vi "ゲージデータ取り込み.vi"(8 "測定周期/ms":dbl, 9 "値転記用配列_\n設定項目画面からの転記":T1[](array[typedef]) {"測定モード" items=["単発測定モード", "連続測定モード", "多点測定モード"]}, 10 "ゲージ確認ボタンBOOL":bool) -> (0 "書込周期/ms":dbl, 11 "実測設定項目配列_\nメインからの転記":T1[](array[typedef]) {"測定モード" items=["単発測定モード", "連続測定モード", "多点測定モード"]})   [LabVIEW 2021]
uses:
  <vilib>/Utility/config.llb/Read Key (U32).vi
  <vilib>/Utility/config.llb/Read Key (String).vi
  <vilib>/Utility/config.llb/Read Key (I32).vi
  <vilib>/Utility/config.llb/Read Key (Boolean).vi
  <vilib>/Utility/config.llb/NI_LVConfig.lvlib
panel:
  out "メイン設定_設定 12":T1 {"測定モード" items=["単発測定モード", "連続測定モード", "多点測定モード"]}
  out "メイン設定_設定 11":T1 {"測定モード" items=["単発測定モード", "連続測定モード", "多点測定モード"]}
  out "メイン設定_設定 10":T1 {"測定モード" items=["単発測定モード", "連続測定モード", "多点測定モード"]}
  out "メイン設定_設定 9":T1 {"測定モード" items=["単発測定モード", "連続測定モード", "多点測定モード"]}
  out "メイン設定_設定 8":T1 {"測定モード" items=["単発測定モード", "連続測定モード", "多点測定モード"]}
  out "メイン設定_設定 7":T1 {"測定モード" items=["単発測定モード", "連続測定モード", "多点測定モード"]}
  out "メイン設定_設定 6":T1 {"測定モード" items=["単発測定モード", "連続測定モード", "多点測定モード"]}
  out "メイン設定_設定 5":T1 {"測定モード" items=["単発測定モード", "連続測定モード", "多点測定モード"]}
  out "メイン設定_設定 4":T1 {"測定モード" items=["単発測定モード", "連続測定モード", "多点測定モード"]}
  out "メイン設定_設定 3":T1 {"測定モード" items=["単発測定モード", "連続測定モード", "多点測定モード"]}
  out "メイン設定_設定 2":T1 {"測定モード" items=["単発測定モード", "連続測定モード", "多点測定モード"]}
  out "メイン設定_設定 1":T1 {"測定モード" items=["単発測定モード", "連続測定モード", "多点測定モード"]}
  out "setup.iniエラーout":errorcluster caption="エラー入力（エラーなし）"
  out "iniフォルダパス取得":path
  in  "setup.iniエラーin":errorcluster caption="エラー入力（エラーなし）"
  out "ゲージエラー 12":errorcluster caption="エラー入力 (エラーなし)"
  out "ゲージエラー 11":errorcluster caption="エラー入力 (エラーなし)"
  out "ゲージエラー 10":errorcluster caption="エラー入力 (エラーなし)"
  out "ゲージエラー 9":errorcluster caption="エラー入力 (エラーなし)"
  out "ゲージエラー 8":errorcluster caption="エラー入力 (エラーなし)"
  out "ゲージエラー 7":errorcluster caption="エラー入力 (エラーなし)"
  out "ゲージエラー 6":errorcluster caption="エラー入力 (エラーなし)"
  out "ゲージエラー 5":errorcluster caption="エラー入力 (エラーなし)"
  out "ゲージエラー 4":errorcluster caption="エラー入力 (エラーなし)"
  out "ゲージエラー 3":errorcluster caption="エラー入力 (エラーなし)"
  out "ゲージエラー 2":errorcluster caption="エラー入力 (エラーなし)"
  out "ゲージエラー 1":errorcluster caption="エラー入力 (エラーなし)"
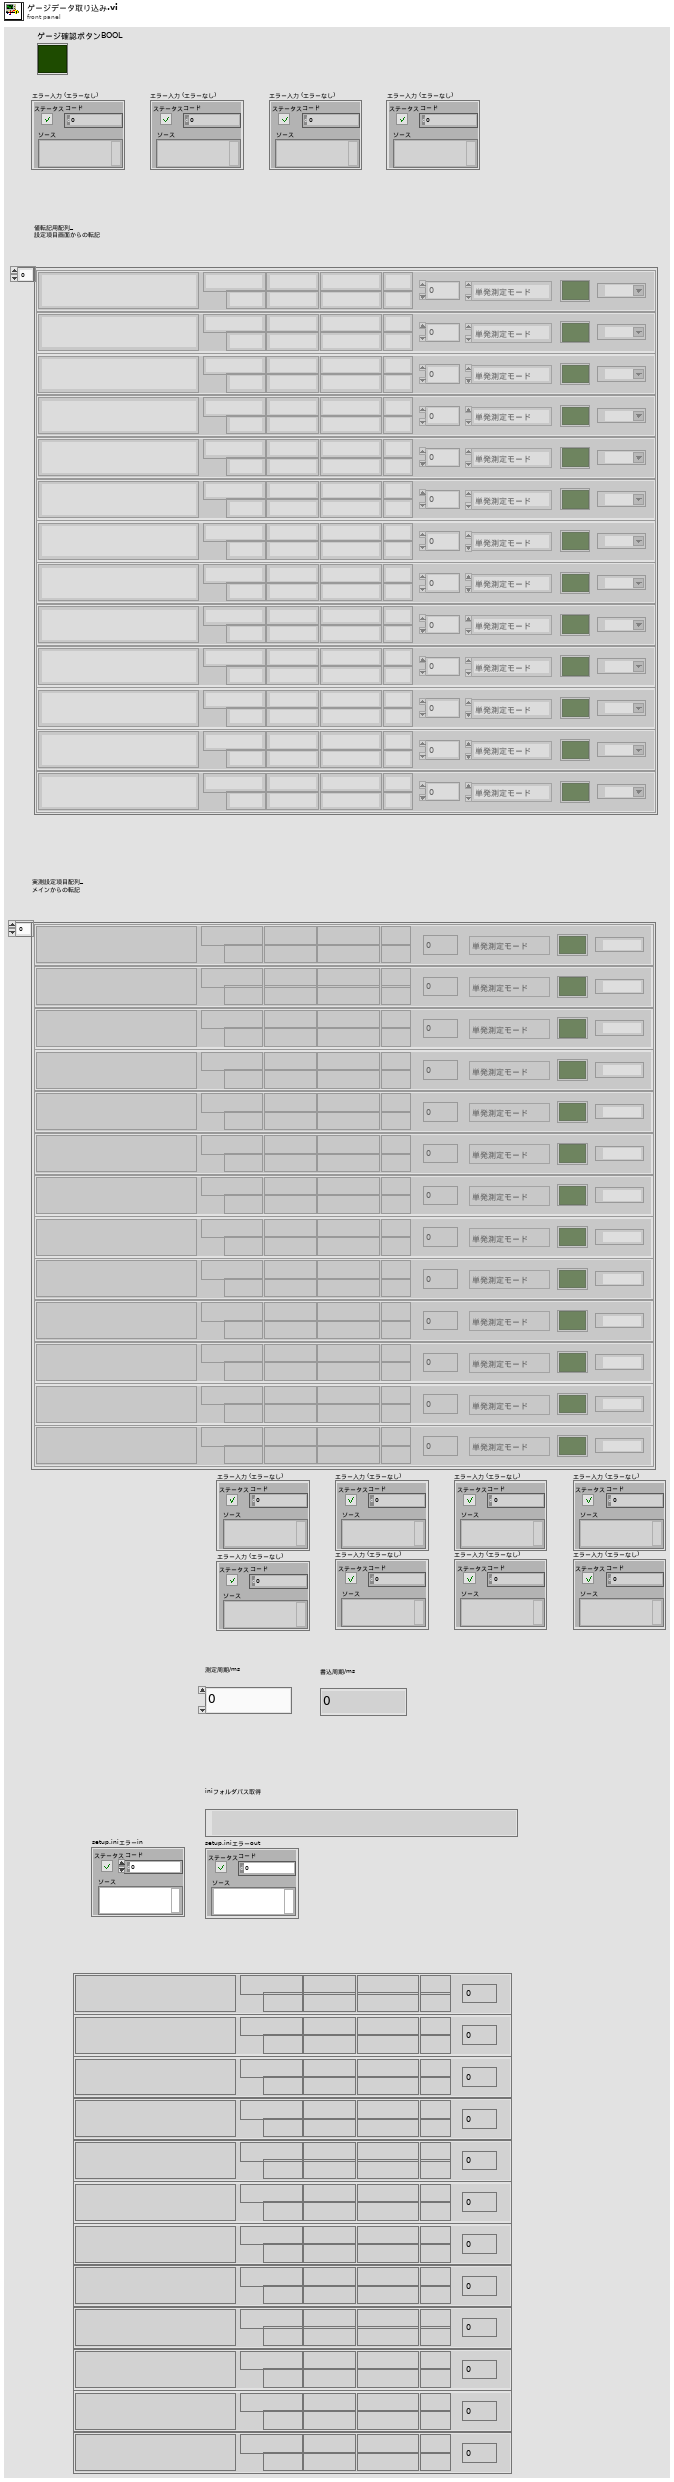
[diagram p1: front panel]
types:
  T1 = typedef "設定全項目制御器.ctl" = cluster{"規格":string, "規格上限":string, "規格下限":string, "ポートNo.":dbl, "測定モード":u16, "規格単位":string, "品質チェック項目":string, "測定周期":dbl, "実測値MAX":string, "実測値MIN":string, "実測値(MAX)":string, "実測値(MIN)":string, "測定画面表示ボタン":bool, "ゲージポートNo":refnum<visa-resource-name>}
  T2 = typedef "NI_LVConfig.lvlib/Config Data RefNum.ctl" = refnum<k1>
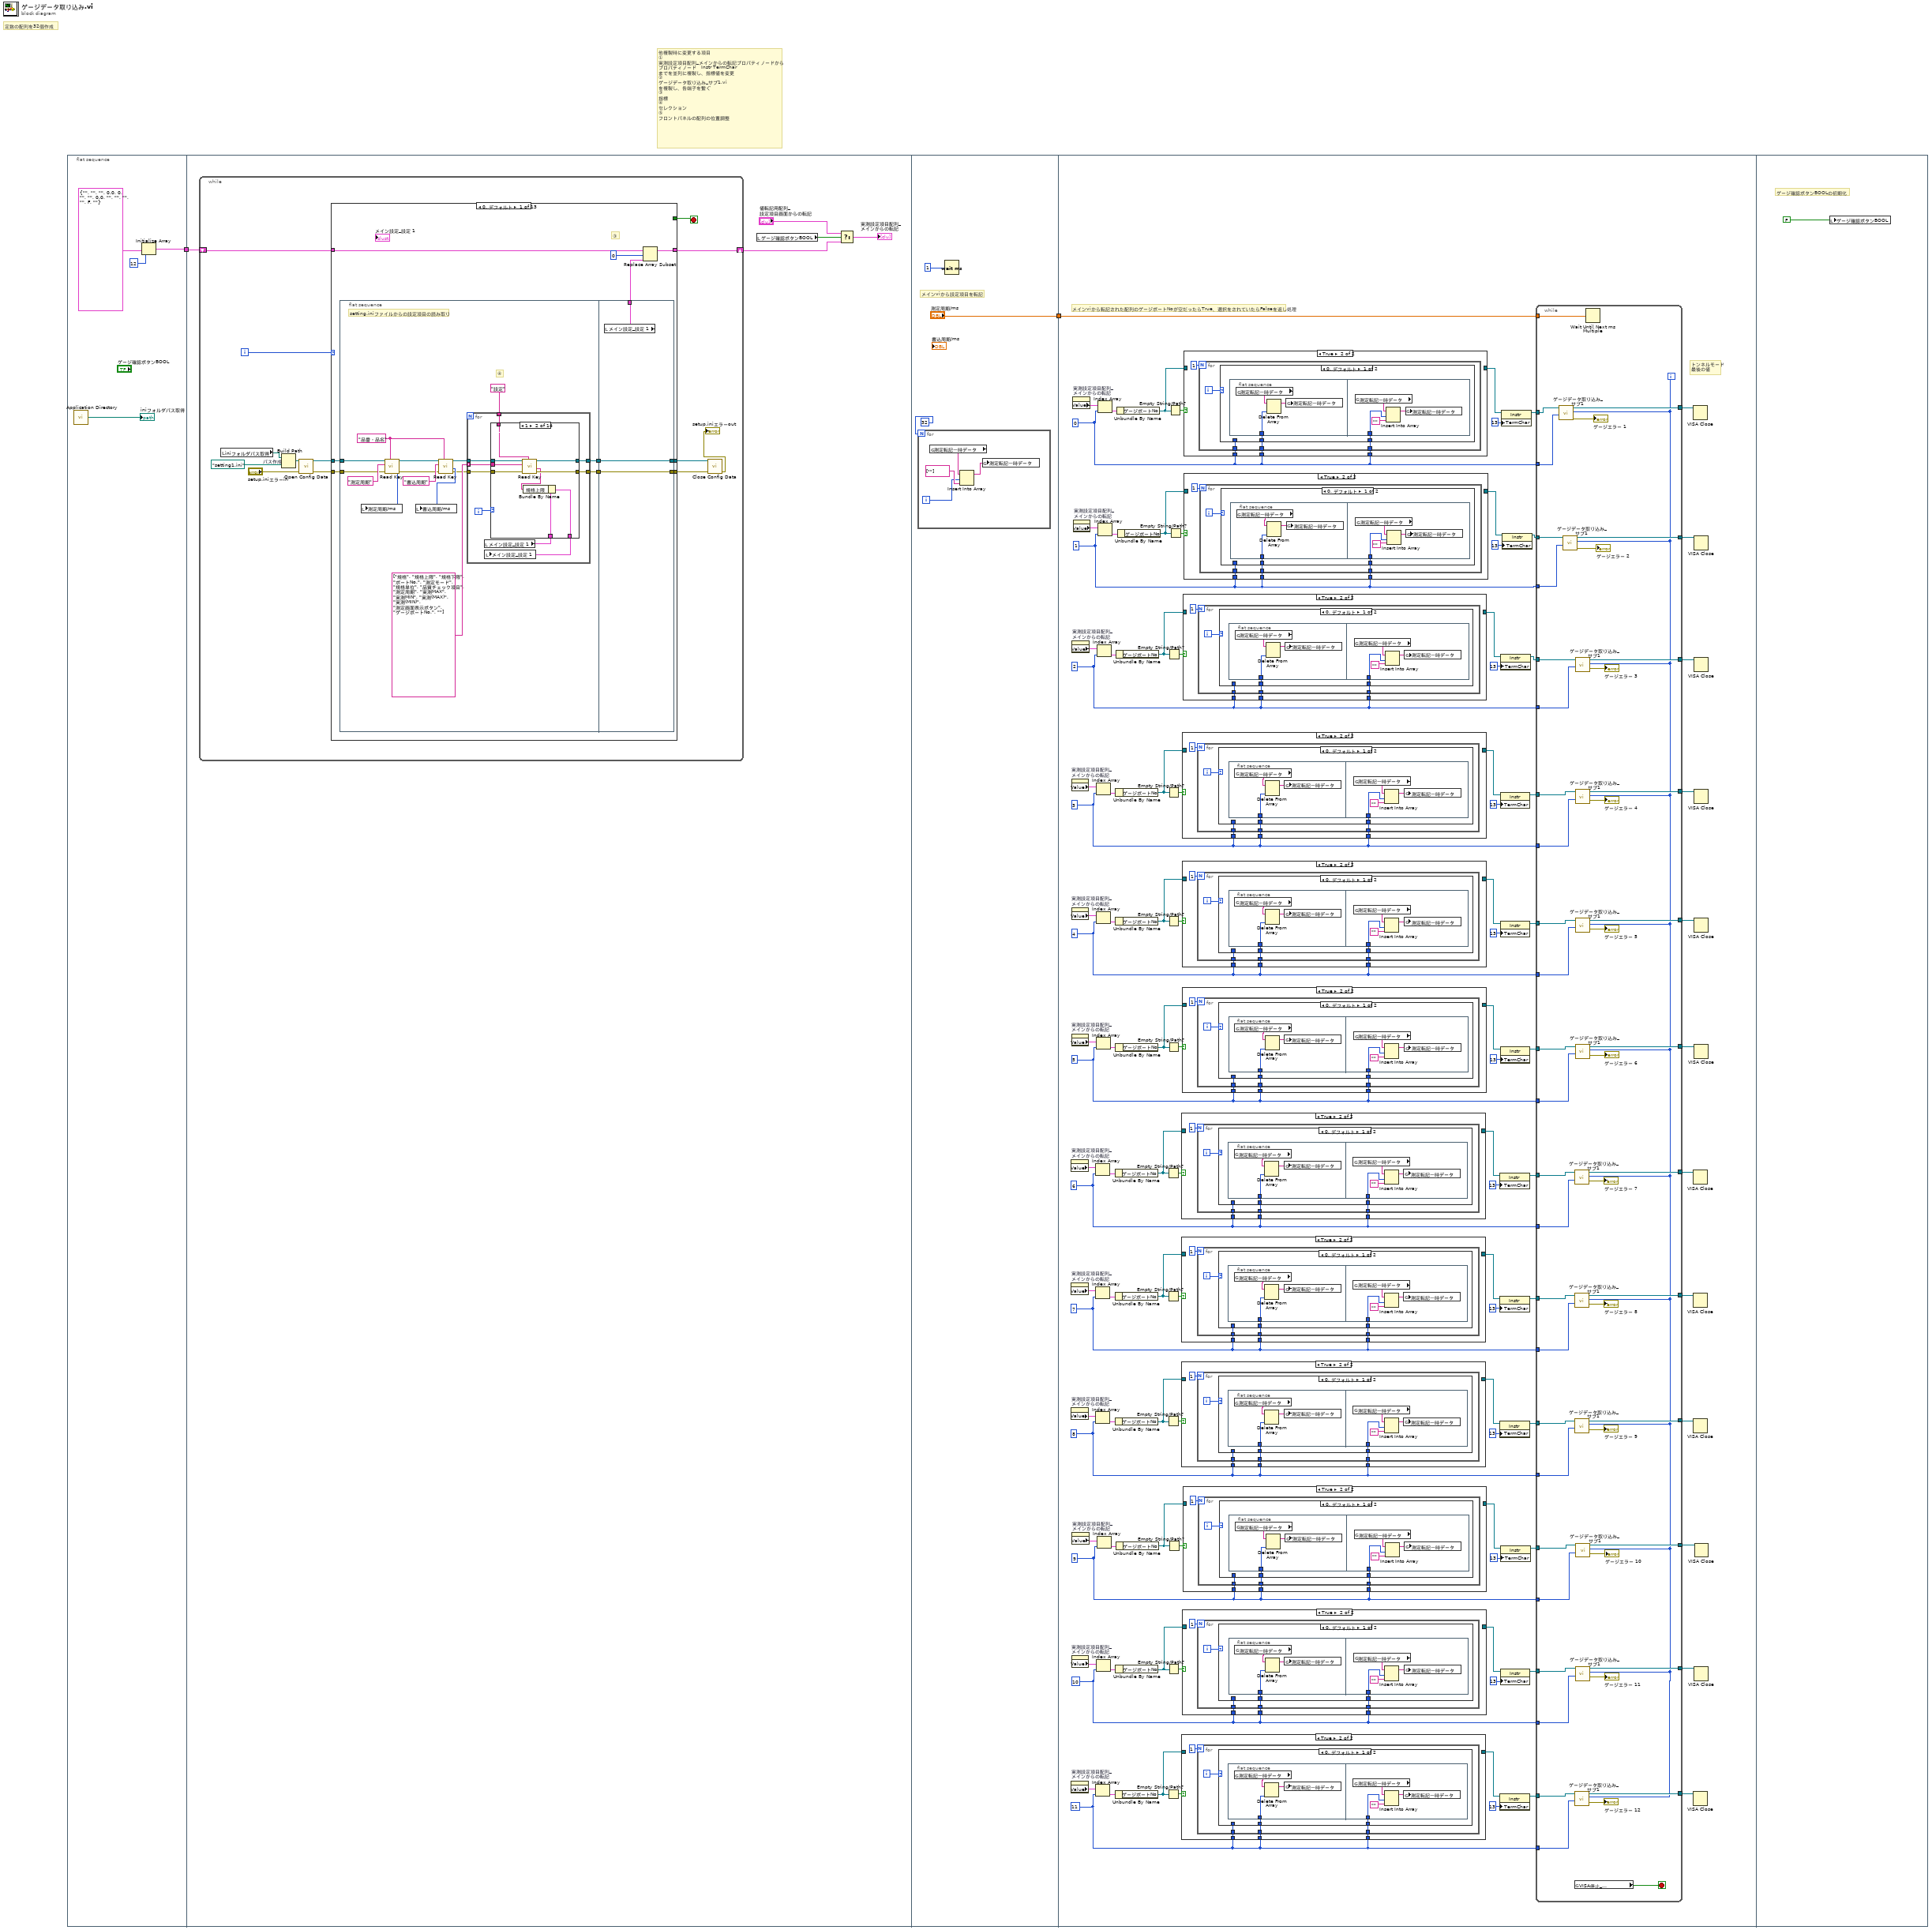
[diagram p0: block diagram]
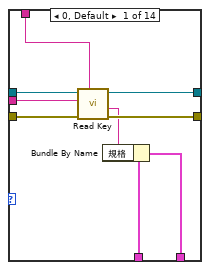
[diagram p2: hidden frame]
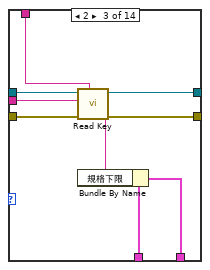
[diagram p3: hidden frame]
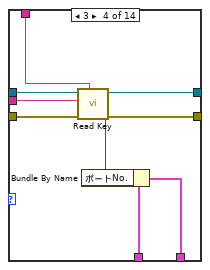
[diagram p4: hidden frame]
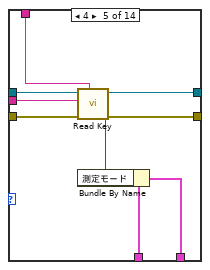
[diagram p5: hidden frame]
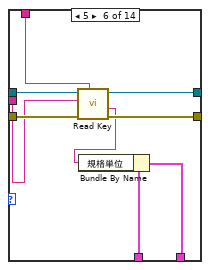
[diagram p6: hidden frame]
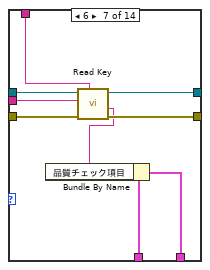
[diagram p7: hidden frame]
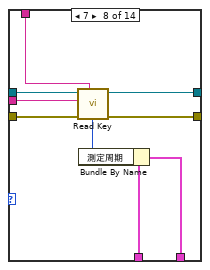
[diagram p8: hidden frame]
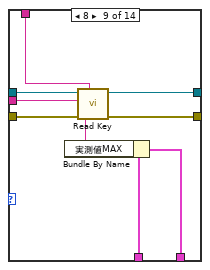
[diagram p9: hidden frame]
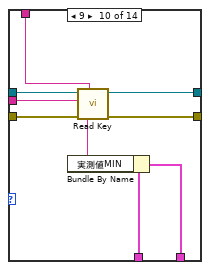
[diagram p10: hidden frame]
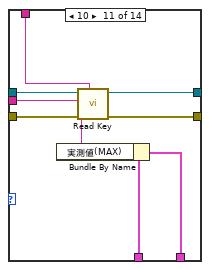
[diagram p11: hidden frame]
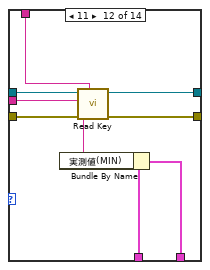
[diagram p12: hidden frame]
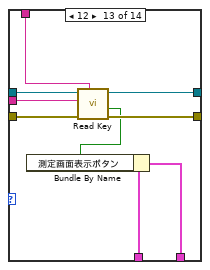
[diagram p13: hidden frame]
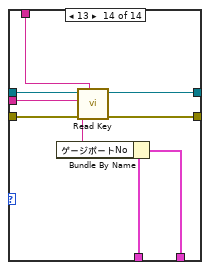
[diagram p14: hidden frame]
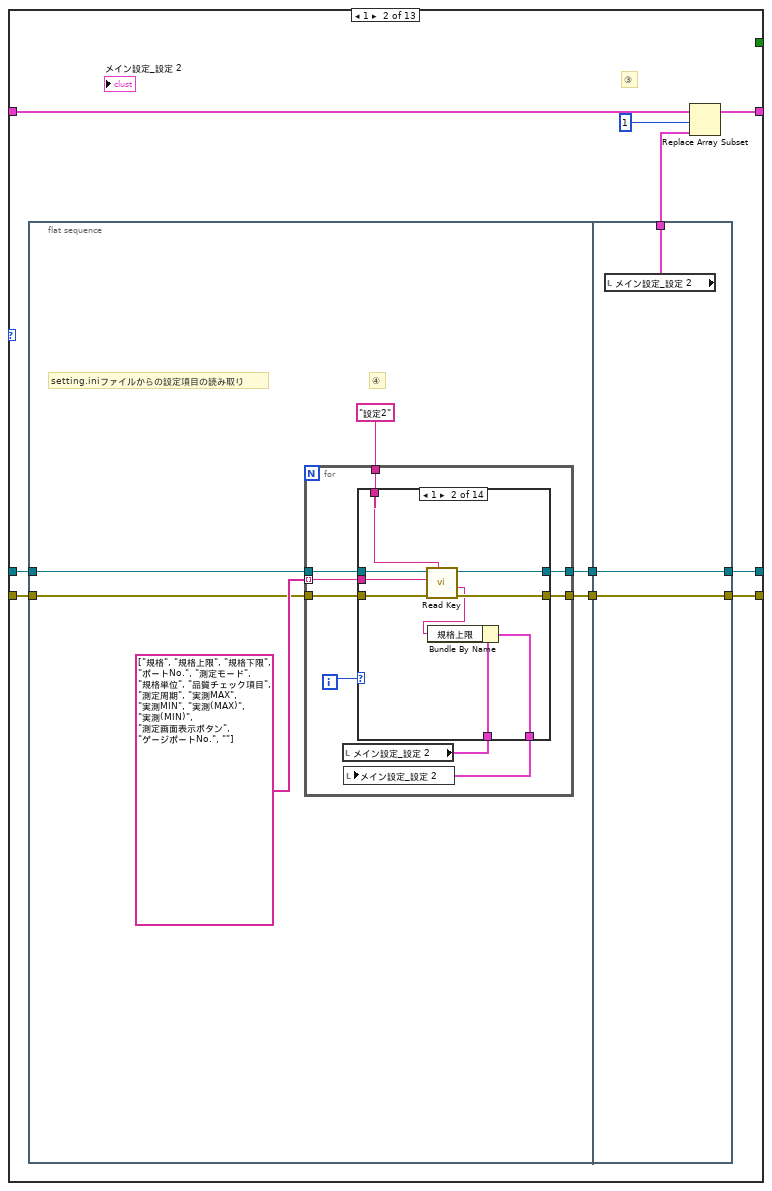
[diagram p15: hidden frame]
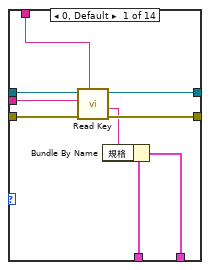
[diagram p16: hidden frame]
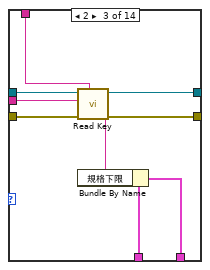
[diagram p17: hidden frame]
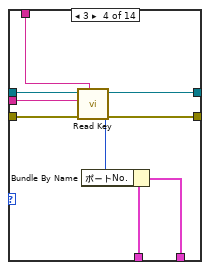
[diagram p18: hidden frame]
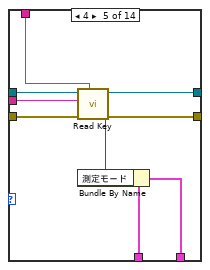
[diagram p19: hidden frame]
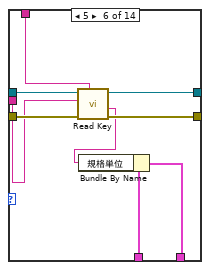
[diagram p20: hidden frame]
diagram:
  # "他複製時に変更する項目\n①\n実測設定項目配列_メインからの転記プロパティノードから\nプロパティノード　Instr TermChar\nまでを並列に複製し、指標値を変更\n②\nゲージデータ取り込み_サブ1.vi\nを複製し、各端子を繋ぐ\n③\n指標\n④\nセレクション\n⑤\nフロントパネルの配列の位置調整"
  # "定数の配列を32個作成"
  n1 = flat-sequence {
    tunnel: [w3] -> w1
    tunnel: w1 -> [w11]
    tunnel: ["測定周期/ms"] -> w2
    tunnel: w2 -> [w1991]
    frame #0 {
      n2 = call <vilib>:"Application Directory.vi"() -> ("Application Directory"=→"iniフォルダパス取得":path)
      n3 = Initialize Array(T1 {"規格"="", "規格上限"="", "規格下限"="", "ポートNo."=0.0, "測定モード"=0, "規格単位"="", "品質チェック項目"="", "測定周期"=0.0, "実測値MAX"="", "実測値MIN"="", "実測値(MAX)"="", "実測値(MIN)"="", "測定画面表示ボタン"=FALSE, "ゲージポートNo"=""} ("メイン設定_設定"), 12) -> (w3:T1[])
    }
    frame #1 {
      n4 = while {
        shift-right: [w12] -> w9
        shift-left: w11 -> [w14]
        i -> [w19]
        stop <- w13 stop-if-true
        n5 = local read "iniフォルダパス取得"() -> (w24:path)
        n6 = Build Path "パス作成"(base path=w24, name or relative path=path "setting1.ini") -> (appended path=w23:path)
        n7 = call <vilib>:"Open Config Data.vi"("error in (no error)"="setup.iniエラーin", "configuration file path"=w23) -> ("error out"=w17:errorcluster, "refnum"=w18:T2)  [unwired: 1 in, 7 out]
        n8 = case shown="0, デフォルト" w19 {
          tunnel: w18 -> [w34 w197 w351 w505 w659 w813 w967 w1121 w1275 w1429 w1583 w1737 w1883]
          tunnel: w17 -> [w33 w196 w350 w504 w658 w812 w966 w1120 w1274 w1428 w1582 w1736 w1882]
          tunnel: [w32 w195 w349 w503 w657 w811 w965 w1119 w1273 w1427 w1581 w1735 w1883] -> w16
          tunnel: [w31 w194 w348 w502 w656 w810 w964 w1118 w1272 w1426 w1580 w1734 w1882] -> w15
          tunnel: w14 -> [w28 w191 w345 w499 w653 w807 w961 w1115 w1269 w1423 w1577 w1731 w1884]
          tunnel: [w27 w190 w344 w498 w652 w806 w960 w1114 w1268 w1422 w1576 w1730 w1884] -> w12
          tunnel: [_ _ _ _ _ _ _ _ _ _ _ _ TRUE] -> w13
          frame 0, Default {
            # "③"
            n9 = flat-sequence {
              tunnel: w34 -> [w43]
              tunnel: w33 -> [w42]
              tunnel: [w49] -> w30
              tunnel: [w48] -> w29
              tunnel: [w186] -> w31
              tunnel: [w187] -> w32
              tunnel: w30 -> [w187]
              tunnel: w29 -> [w186]
              tunnel: [w185] -> w26
              frame #0 {
                w41 = "品番・品名"
                # "④"
                # "setting.iniファイルからの設定項目の読み取り"
                n10 = call-poly <vilib>:"Read Key.vi"("section"=w41, "error in (no error)"=w42, "key"="測定周期", "refnum"=w43) -> ("error out"=w38:errorcluster, "value"=w44:u32, "refnum out"=w39:T2)  [unwired: 4 in, 1 out]
                n11 = local write "測定周期/ms"(w44) -> ()
                n12 = call-poly <vilib>:"Read Key.vi"("section"=w41, "error in (no error)"=w38, "key"="書込周期", "refnum"=w39) -> ("error out"=w35:errorcluster, "value"=w37:u32, "refnum out"=w36:T2)  [unwired: 4 in, 1 out]
                n13 = local write "書込周期/ms"(w37) -> ()
                n14 = for {
                  tunnel: "設定" -> [w57]
                  tunnel: string[] ["規格", "規格上限", "規格下限", "ポートNo.", "測定モード", "規格単位", "品質チェック項目", "測定周期", "実測MAX", "実測MIN", "実測(MAX)", "実測(MIN)", "測定画面表示ボタン", "ゲージポートNo.", ""] -> [w52] mode=indexing
                  tunnel: w35 -> [w54]
                  tunnel: [w53] -> w48
                  tunnel: w36 -> [w58]
                  tunnel: [w56] -> w49
                  i -> [w55]
                  n15 = local read "メイン設定_設定 1"() -> (w50:T1)
                  n16 = case shown="1" w55 {
                    tunnel: w58 -> [w67 w76 w85 w94 w103 w112 w121 w130 w139 w148 w157 w166 w175 w184]
                    tunnel: [w66 w75 w84 w93 w102 w111 w120 w129 w138 w147 w156 w165 w174 w183] -> w56
                    tunnel: w57 -> [w65 w74 w83 w92 w101 w110 w119 w128 w137 w146 w155 w164 w173 w182]
                    tunnel: w54 -> [w64 w73 w82 w91 w100 w109 w118 w127 w136 w145 w154 w163 w172 w181]
                    tunnel: [w63 w72 w81 w90 w99 w108 w117 w126 w135 w144 w153 w162 w171 w180] -> w53
                    tunnel: w52 -> [w61 w70 w79 w88 w97 w106 w115 w124 w133 w142 w151 w160 w169 w178]
                    tunnel: [w60 w69 w78 w87 w96 w104 w113 w122 w132 w141 w150 w159 w168 w177] -> w51
                    tunnel: w50 -> [w59 w68 w77 w86 w95 w105 w114 w123 w131 w140 w149 w158 w167 w176]
                    frame 0, Default {
                      n17 = call-poly <vilib>:"Read Key.vi"("section"=w65, "error in (no error)"=w64, "key"=w61, "refnum"=w67) -> ("error out"=w63:errorcluster, "value"=w62:string, "refnum out"=w66:T2)  [unwired: 4 in, 1 out]
                      n18 = Bundle By Name(cluster=w59, "規格"=w62) -> (w60:T1)
                    }
                    frame 1 {
                      n19 = call-poly <vilib>:"Read Key.vi"("section"=w74, "error in (no error)"=w73, "key"=w70, "refnum"=w76) -> ("error out"=w72:errorcluster, "value"=w71:string, "refnum out"=w75:T2)  [unwired: 4 in, 1 out]
                      n20 = Bundle By Name(cluster=w68, "規格上限"=w71) -> (w69:T1)
                    }
                    frame 2 {
                      n21 = call-poly <vilib>:"Read Key.vi"("section"=w83, "error in (no error)"=w82, "key"=w79, "refnum"=w85) -> ("error out"=w81:errorcluster, "value"=w80:string, "refnum out"=w84:T2)  [unwired: 4 in, 1 out]
                      n22 = Bundle By Name(cluster=w77, "規格下限"=w80) -> (w78:T1)
                    }
                    frame 3 {
                      n23 = call-poly <vilib>:"Read Key.vi"("section"=w92, "error in (no error)"=w91, "key"=w88, "refnum"=w94) -> ("error out"=w90:errorcluster, "value"=w89:i32, "refnum out"=w93:T2)  [unwired: 4 in, 1 out]
                      n24 = Bundle By Name(cluster=w86, "ポートNo."=w89) -> (w87:T1)
                    }
                    frame 4 {
                      n25 = call-poly <vilib>:"Read Key.vi"("section"=w101, "error in (no error)"=w100, "key"=w97, "refnum"=w103) -> ("error out"=w99:errorcluster, "value"=w98:i32, "refnum out"=w102:T2)  [unwired: 4 in, 1 out]
                      n26 = Bundle By Name(cluster=w95, "測定モード"=w98) -> (w96:T1)
                    }
                    frame 5 {
                      n27 = call-poly <vilib>:"Read Key.vi"("section"=w110, "error in (no error)"=w109, "key"=w106, "refnum"=w112) -> ("error out"=w108:errorcluster, "value"=w107:string, "refnum out"=w111:T2)  [unwired: 4 in, 1 out]
                      n28 = Bundle By Name(cluster=w105, "規格単位"=w107) -> (w104:T1)
                    }
                    frame 6 {
                      n29 = call-poly <vilib>:"Read Key.vi"("section"=w119, "error in (no error)"=w118, "key"=w115, "refnum"=w121) -> ("error out"=w117:errorcluster, "value"=w116:string, "refnum out"=w120:T2)  [unwired: 4 in, 1 out]
                      n30 = Bundle By Name(cluster=w114, "品質チェック項目"=w116) -> (w113:T1)
                    }
                    frame 7 {
                      n31 = call-poly <vilib>:"Read Key.vi"("section"=w128, "error in (no error)"=w127, "key"=w124, "refnum"=w130) -> ("error out"=w126:errorcluster, "value"=w125:i32, "refnum out"=w129:T2)  [unwired: 4 in, 1 out]
                      n32 = Bundle By Name(cluster=w123, "測定周期"=w125) -> (w122:T1)
                    }
                    frame 8 {
                      n33 = call-poly <vilib>:"Read Key.vi"("section"=w137, "error in (no error)"=w136, "key"=w133, "refnum"=w139) -> ("error out"=w135:errorcluster, "value"=w134:string, "refnum out"=w138:T2)  [unwired: 4 in, 1 out]
                      n34 = Bundle By Name(cluster=w131, "実測値MAX"=w134) -> (w132:T1)
                    }
                    frame 9 {
                      n35 = call-poly <vilib>:"Read Key.vi"("section"=w146, "error in (no error)"=w145, "key"=w142, "refnum"=w148) -> ("error out"=w144:errorcluster, "value"=w143:string, "refnum out"=w147:T2)  [unwired: 4 in, 1 out]
                      n36 = Bundle By Name(cluster=w140, "実測値MIN"=w143) -> (w141:T1)
                    }
                    frame 10 {
                      n37 = call-poly <vilib>:"Read Key.vi"("section"=w155, "error in (no error)"=w154, "key"=w151, "refnum"=w157) -> ("error out"=w153:errorcluster, "value"=w152:string, "refnum out"=w156:T2)  [unwired: 4 in, 1 out]
                      n38 = Bundle By Name(cluster=w149, "実測値(MAX)"=w152) -> (w150:T1)
                    }
                    frame 11 {
                      n39 = call-poly <vilib>:"Read Key.vi"("section"=w164, "error in (no error)"=w163, "key"=w160, "refnum"=w166) -> ("error out"=w162:errorcluster, "value"=w161:string, "refnum out"=w165:T2)  [unwired: 4 in, 1 out]
                      n40 = Bundle By Name(cluster=w158, "実測値(MIN)"=w161) -> (w159:T1)
                    }
                    frame 12 {
                      n41 = call-poly <vilib>:"Read Key.vi"("section"=w173, "error in (no error)"=w172, "key"=w169, "refnum"=w175) -> ("error out"=w171:errorcluster, "value"=w170:bool, "refnum out"=w174:T2)  [unwired: 4 in, 1 out]
                      n42 = Bundle By Name(cluster=w167, "測定画面表示ボタン"=w170) -> (w168:T1)
                    }
                    frame 13 {
                      n43 = call-poly <vilib>:"Read Key.vi"("section"=w182, "error in (no error)"=w181, "key"=w178, "refnum"=w184) -> ("error out"=w180:errorcluster, "value"=w179:string, "refnum out"=w183:T2)  [unwired: 4 in, 1 out]
                      n44 = Bundle By Name(cluster=w176, "ゲージポートNo"=w179) -> (w177:T1)
                    }
                  }
                  n45 = local write "メイン設定_設定 1"(w51) -> ()
                }
              }
              frame #1 {
                n46 = local read "メイン設定_設定 1"() -> (w185:T1)
              }
            }
            n47 = Replace Array Subset(array=w28, new element=w26, index=0) -> (w27:T1[])
          }
          frame 1 {
            # "③"
            n48 = flat-sequence {
              tunnel: w197 -> [w199]
              tunnel: w196 -> [w198]
              tunnel: [w203] -> w193
              tunnel: [w202] -> w192
              tunnel: [w340] -> w194
              tunnel: [w341] -> w195
              tunnel: w193 -> [w341]
              tunnel: w192 -> [w340]
              tunnel: [w339] -> w189
              frame #0 {
                # "④"
                # "setting.iniファイルからの設定項目の読み取り"
                n49 = for {
                  tunnel: "設定2" -> [w211]
                  tunnel: string[] ["規格", "規格上限", "規格下限", "ポートNo.", "測定モード", "規格単位", "品質チェック項目", "測定周期", "実測MAX", "実測MIN", "実測(MAX)", "実測(MIN)", "測定画面表示ボタン", "ゲージポートNo.", ""] -> [w206] mode=indexing
                  tunnel: w198 -> [w208]
                  tunnel: [w207] -> w202
                  tunnel: w199 -> [w212]
                  tunnel: [w210] -> w203
                  i -> [w209]
                  n50 = local read "メイン設定_設定 2"() -> (w204:T1)
                  n51 = case shown="1" w209 {
                    tunnel: w212 -> [w221 w230 w239 w248 w257 w266 w275 w284 w293 w302 w311 w320 w329 w338]
                    tunnel: [w220 w229 w238 w247 w256 w265 w274 w283 w292 w301 w310 w319 w328 w337] -> w210
                    tunnel: w211 -> [w219 w228 w237 w246 w255 w264 w273 w282 w291 w300 w309 w318 w327 w336]
                    tunnel: w208 -> [w218 w227 w236 w245 w254 w263 w272 w281 w290 w299 w308 w317 w326 w335]
                    tunnel: [w217 w226 w235 w244 w253 w262 w271 w280 w289 w298 w307 w316 w325 w334] -> w207
                    tunnel: w206 -> [w215 w224 w233 w242 w251 w260 w269 w278 w287 w296 w305 w314 w323 w332]
                    tunnel: [w214 w223 w232 w241 w250 w258 w267 w276 w286 w295 w304 w313 w322 w331] -> w205
                    tunnel: w204 -> [w213 w222 w231 w240 w249 w259 w268 w277 w285 w294 w303 w312 w321 w330]
                    frame 0, Default {
                      n52 = call-poly <vilib>:"Read Key.vi"("section"=w219, "error in (no error)"=w218, "key"=w215, "refnum"=w221) -> ("error out"=w217:errorcluster, "value"=w216:string, "refnum out"=w220:T2)  [unwired: 4 in, 1 out]
                      n53 = Bundle By Name(cluster=w213, "規格"=w216) -> (w214:T1)
                    }
                    frame 1 {
                      n54 = call-poly <vilib>:"Read Key.vi"("section"=w228, "error in (no error)"=w227, "key"=w224, "refnum"=w230) -> ("error out"=w226:errorcluster, "value"=w225:string, "refnum out"=w229:T2)  [unwired: 4 in, 1 out]
                      n55 = Bundle By Name(cluster=w222, "規格上限"=w225) -> (w223:T1)
                    }
                    frame 2 {
                      n56 = call-poly <vilib>:"Read Key.vi"("section"=w237, "error in (no error)"=w236, "key"=w233, "refnum"=w239) -> ("error out"=w235:errorcluster, "value"=w234:string, "refnum out"=w238:T2)  [unwired: 4 in, 1 out]
                      n57 = Bundle By Name(cluster=w231, "規格下限"=w234) -> (w232:T1)
                    }
                    frame 3 {
                      n58 = call-poly <vilib>:"Read Key.vi"("section"=w246, "error in (no error)"=w245, "key"=w242, "refnum"=w248) -> ("error out"=w244:errorcluster, "value"=w243:i32, "refnum out"=w247:T2)  [unwired: 4 in, 1 out]
                      n59 = Bundle By Name(cluster=w240, "ポートNo."=w243) -> (w241:T1)
                    }
                    frame 4 {
                      n60 = call-poly <vilib>:"Read Key.vi"("section"=w255, "error in (no error)"=w254, "key"=w251, "refnum"=w257) -> ("error out"=w253:errorcluster, "value"=w252:i32, "refnum out"=w256:T2)  [unwired: 4 in, 1 out]
                      n61 = Bundle By Name(cluster=w249, "測定モード"=w252) -> (w250:T1)
                    }
                    frame 5 {
                      n62 = call-poly <vilib>:"Read Key.vi"("section"=w264, "error in (no error)"=w263, "key"=w260, "refnum"=w266) -> ("error out"=w262:errorcluster, "value"=w261:string, "refnum out"=w265:T2)  [unwired: 4 in, 1 out]
                      n63 = Bundle By Name(cluster=w259, "規格単位"=w261) -> (w258:T1)
                    }
                    frame 6 {
                      n64 = call-poly <vilib>:"Read Key.vi"("section"=w273, "error in (no error)"=w272, "key"=w269, "refnum"=w275) -> ("error out"=w271:errorcluster, "value"=w270:string, "refnum out"=w274:T2)  [unwired: 4 in, 1 out]
                      n65 = Bundle By Name(cluster=w268, "品質チェック項目"=w270) -> (w267:T1)
                    }
                    frame 7 {
                      n66 = call-poly <vilib>:"Read Key.vi"("section"=w282, "error in (no error)"=w281, "key"=w278, "refnum"=w284) -> ("error out"=w280:errorcluster, "value"=w279:i32, "refnum out"=w283:T2)  [unwired: 4 in, 1 out]
                      n67 = Bundle By Name(cluster=w277, "測定周期"=w279) -> (w276:T1)
                    }
                    frame 8 {
                      n68 = call-poly <vilib>:"Read Key.vi"("section"=w291, "error in (no error)"=w290, "key"=w287, "refnum"=w293) -> ("error out"=w289:errorcluster, "value"=w288:string, "refnum out"=w292:T2)  [unwired: 4 in, 1 out]
                      n69 = Bundle By Name(cluster=w285, "実測値MAX"=w288) -> (w286:T1)
                    }
                    frame 9 {
                      n70 = call-poly <vilib>:"Read Key.vi"("section"=w300, "error in (no error)"=w299, "key"=w296, "refnum"=w302) -> ("error out"=w298:errorcluster, "value"=w297:string, "refnum out"=w301:T2)  [unwired: 4 in, 1 out]
                      n71 = Bundle By Name(cluster=w294, "実測値MIN"=w297) -> (w295:T1)
                    }
                    frame 10 {
                      n72 = call-poly <vilib>:"Read Key.vi"("section"=w309, "error in (no error)"=w308, "key"=w305, "refnum"=w311) -> ("error out"=w307:errorcluster, "value"=w306:string, "refnum out"=w310:T2)  [unwired: 4 in, 1 out]
                      n73 = Bundle By Name(cluster=w303, "実測値(MAX)"=w306) -> (w304:T1)
                    }
                    frame 11 {
                      n74 = call-poly <vilib>:"Read Key.vi"("section"=w318, "error in (no error)"=w317, "key"=w314, "refnum"=w320) -> ("error out"=w316:errorcluster, "value"=w315:string, "refnum out"=w319:T2)  [unwired: 4 in, 1 out]
                      n75 = Bundle By Name(cluster=w312, "実測値(MIN)"=w315) -> (w313:T1)
                    }
                    frame 12 {
                      n76 = call-poly <vilib>:"Read Key.vi"("section"=w327, "error in (no error)"=w326, "key"=w323, "refnum"=w329) -> ("error out"=w325:errorcluster, "value"=w324:bool, "refnum out"=w328:T2)  [unwired: 4 in, 1 out]
                      n77 = Bundle By Name(cluster=w321, "測定画面表示ボタン"=w324) -> (w322:T1)
                    }
                    frame 13 {
                      n78 = call-poly <vilib>:"Read Key.vi"("section"=w336, "error in (no error)"=w335, "key"=w332, "refnum"=w338) -> ("error out"=w334:errorcluster, "value"=w333:string, "refnum out"=w337:T2)  [unwired: 4 in, 1 out]
                      n79 = Bundle By Name(cluster=w330, "ゲージポートNo"=w333) -> (w331:T1)
                    }
                  }
                  n80 = local write "メイン設定_設定 2"(w205) -> ()
                }
              }
              frame #1 {
                n81 = local read "メイン設定_設定 2"() -> (w339:T1)
              }
            }
            n82 = Replace Array Subset(array=w191, new element=w189, index=1) -> (w190:T1[])
          }
          frame 2 {
            # "③"
            n83 = flat-sequence {
              tunnel: w351 -> [w353]
              tunnel: w350 -> [w352]
              tunnel: [w357] -> w347
              tunnel: [w356] -> w346
              tunnel: [w494] -> w348
              tunnel: [w495] -> w349
              tunnel: w347 -> [w495]
              tunnel: w346 -> [w494]
              tunnel: [w493] -> w343
              frame #0 {
                # "④"
                # "setting.iniファイルからの設定項目の読み取り"
                n84 = for {
                  tunnel: "設定3" -> [w365]
                  tunnel: string[] ["規格", "規格上限", "規格下限", "ポートNo.", "測定モード", "規格単位", "品質チェック項目", "測定周期", "実測MAX", "実測MIN", "実測(MAX)", "実測(MIN)", "測定画面表示ボタン", "ゲージポートNo.", ""] -> [w360] mode=indexing
                  tunnel: w352 -> [w362]
                  tunnel: [w361] -> w356
                  tunnel: w353 -> [w366]
                  tunnel: [w364] -> w357
                  i -> [w363]
                  n85 = local read "メイン設定_設定 3"() -> (w358:T1)
                  n86 = case shown="1" w363 {
                    tunnel: w366 -> [w375 w384 w393 w402 w411 w420 w429 w438 w447 w456 w465 w474 w483 w492]
                    tunnel: [w374 w383 w392 w401 w410 w419 w428 w437 w446 w455 w464 w473 w482 w491] -> w364
                    tunnel: w365 -> [w373 w382 w391 w400 w409 w418 w427 w436 w445 w454 w463 w472 w481 w490]
                    tunnel: w362 -> [w372 w381 w390 w399 w408 w417 w426 w435 w444 w453 w462 w471 w480 w489]
                    tunnel: [w371 w380 w389 w398 w407 w416 w425 w434 w443 w452 w461 w470 w479 w488] -> w361
                    tunnel: w360 -> [w369 w378 w387 w396 w405 w414 w423 w432 w441 w450 w459 w468 w477 w486]
                    tunnel: [w368 w377 w386 w395 w404 w412 w421 w430 w440 w449 w458 w467 w476 w485] -> w359
                    tunnel: w358 -> [w367 w376 w385 w394 w403 w413 w422 w431 w439 w448 w457 w466 w475 w484]
                    frame 0, Default {
                      n87 = call-poly <vilib>:"Read Key.vi"("section"=w373, "error in (no error)"=w372, "key"=w369, "refnum"=w375) -> ("error out"=w371:errorcluster, "value"=w370:string, "refnum out"=w374:T2)  [unwired: 4 in, 1 out]
                      n88 = Bundle By Name(cluster=w367, "規格"=w370) -> (w368:T1)
                    }
                    frame 1 {
                      n89 = call-poly <vilib>:"Read Key.vi"("section"=w382, "error in (no error)"=w381, "key"=w378, "refnum"=w384) -> ("error out"=w380:errorcluster, "value"=w379:string, "refnum out"=w383:T2)  [unwired: 4 in, 1 out]
                      n90 = Bundle By Name(cluster=w376, "規格上限"=w379) -> (w377:T1)
                    }
                    frame 2 {
                      n91 = call-poly <vilib>:"Read Key.vi"("section"=w391, "error in (no error)"=w390, "key"=w387, "refnum"=w393) -> ("error out"=w389:errorcluster, "value"=w388:string, "refnum out"=w392:T2)  [unwired: 4 in, 1 out]
                      n92 = Bundle By Name(cluster=w385, "規格下限"=w388) -> (w386:T1)
                    }
                    frame 3 {
                      n93 = call-poly <vilib>:"Read Key.vi"("section"=w400, "error in (no error)"=w399, "key"=w396, "refnum"=w402) -> ("error out"=w398:errorcluster, "value"=w397:i32, "refnum out"=w401:T2)  [unwired: 4 in, 1 out]
                      n94 = Bundle By Name(cluster=w394, "ポートNo."=w397) -> (w395:T1)
                    }
                    frame 4 {
                      n95 = call-poly <vilib>:"Read Key.vi"("section"=w409, "error in (no error)"=w408, "key"=w405, "refnum"=w411) -> ("error out"=w407:errorcluster, "value"=w406:i32, "refnum out"=w410:T2)  [unwired: 4 in, 1 out]
                      n96 = Bundle By Name(cluster=w403, "測定モード"=w406) -> (w404:T1)
                    }
                    frame 5 {
                      n97 = call-poly <vilib>:"Read Key.vi"("section"=w418, "error in (no error)"=w417, "key"=w414, "refnum"=w420) -> ("error out"=w416:errorcluster, "value"=w415:string, "refnum out"=w419:T2)  [unwired: 4 in, 1 out]
                      n98 = Bundle By Name(cluster=w413, "規格単位"=w415) -> (w412:T1)
                    }
                    frame 6 {
                      n99 = call-poly <vilib>:"Read Key.vi"("section"=w427, "error in (no error)"=w426, "key"=w423, "refnum"=w429) -> ("error out"=w425:errorcluster, "value"=w424:string, "refnum out"=w428:T2)  [unwired: 4 in, 1 out]
                      n100 = Bundle By Name(cluster=w422, "品質チェック項目"=w424) -> (w421:T1)
                    }
                    frame 7 {
                      n101 = call-poly <vilib>:"Read Key.vi"("section"=w436, "error in (no error)"=w435, "key"=w432, "refnum"=w438) -> ("error out"=w434:errorcluster, "value"=w433:i32, "refnum out"=w437:T2)  [unwired: 4 in, 1 out]
                      n102 = Bundle By Name(cluster=w431, "測定周期"=w433) -> (w430:T1)
                    }
                    frame 8 {
                      n103 = call-poly <vilib>:"Read Key.vi"("section"=w445, "error in (no error)"=w444, "key"=w441, "refnum"=w447) -> ("error out"=w443:errorcluster, "value"=w442:string, "refnum out"=w446:T2)  [unwired: 4 in, 1 out]
                      n104 = Bundle By Name(cluster=w439, "実測値MAX"=w442) -> (w440:T1)
                    }
                    frame 9 {
                      n105 = call-poly <vilib>:"Read Key.vi"("section"=w454, "error in (no error)"=w453, "key"=w450, "refnum"=w456) -> ("error out"=w452:errorcluster, "value"=w451:string, "refnum out"=w455:T2)  [unwired: 4 in, 1 out]
                      n106 = Bundle By Name(cluster=w448, "実測値MIN"=w451) -> (w449:T1)
                    }
                    frame 10 {
                      n107 = call-poly <vilib>:"Read Key.vi"("section"=w463, "error in (no error)"=w462, "key"=w459, "refnum"=w465) -> ("error out"=w461:errorcluster, "value"=w460:string, "refnum out"=w464:T2)  [unwired: 4 in, 1 out]
                      n108 = Bundle By Name(cluster=w457, "実測値(MAX)"=w460) -> (w458:T1)
                    }
                    frame 11 {
                      n109 = call-poly <vilib>:"Read Key.vi"("section"=w472, "error in (no error)"=w471, "key"=w468, "refnum"=w474) -> ("error out"=w470:errorcluster, "value"=w469:string, "refnum out"=w473:T2)  [unwired: 4 in, 1 out]
                      n110 = Bundle By Name(cluster=w466, "実測値(MIN)"=w469) -> (w467:T1)
                    }
                    frame 12 {
                      n111 = call-poly <vilib>:"Read Key.vi"("section"=w481, "error in (no error)"=w480, "key"=w477, "refnum"=w483) -> ("error out"=w479:errorcluster, "value"=w478:bool, "refnum out"=w482:T2)  [unwired: 4 in, 1 out]
                      n112 = Bundle By Name(cluster=w475, "測定画面表示ボタン"=w478) -> (w476:T1)
                    }
                    frame 13 {
                      n113 = call-poly <vilib>:"Read Key.vi"("section"=w490, "error in (no error)"=w489, "key"=w486, "refnum"=w492) -> ("error out"=w488:errorcluster, "value"=w487:string, "refnum out"=w491:T2)  [unwired: 4 in, 1 out]
                      n114 = Bundle By Name(cluster=w484, "ゲージポートNo"=w487) -> (w485:T1)
                    }
                  }
                  n115 = local write "メイン設定_設定 3"(w359) -> ()
                }
              }
              frame #1 {
                n116 = local read "メイン設定_設定 3"() -> (w493:T1)
              }
            }
            n117 = Replace Array Subset(array=w345, new element=w343, index=2) -> (w344:T1[])
          }
          frame 3 {
            # "③"
            n118 = flat-sequence {
              tunnel: w505 -> [w507]
              tunnel: w504 -> [w506]
              tunnel: [w511] -> w501
              tunnel: [w510] -> w500
              tunnel: [w648] -> w502
              tunnel: [w649] -> w503
              tunnel: w501 -> [w649]
              tunnel: w500 -> [w648]
              tunnel: [w647] -> w497
              frame #0 {
                # "④"
                # "setting.iniファイルからの設定項目の読み取り"
                n119 = for {
                  tunnel: "設定4" -> [w519]
                  tunnel: string[] ["規格", "規格上限", "規格下限", "ポートNo.", "測定モード", "規格単位", "品質チェック項目", "測定周期", "実測MAX", "実測MIN", "実測(MAX)", "実測(MIN)", "測定画面表示ボタン", "ゲージポートNo.", ""] -> [w514] mode=indexing
                  tunnel: w506 -> [w516]
                  tunnel: [w515] -> w510
                  tunnel: w507 -> [w520]
                  tunnel: [w518] -> w511
                  i -> [w517]
                  n120 = local read "メイン設定_設定 4"() -> (w512:T1)
                  n121 = case shown="1" w517 {
                    tunnel: w520 -> [w529 w538 w547 w556 w565 w574 w583 w592 w601 w610 w619 w628 w637 w646]
                    tunnel: [w528 w537 w546 w555 w564 w573 w582 w591 w600 w609 w618 w627 w636 w645] -> w518
                    tunnel: w519 -> [w527 w536 w545 w554 w563 w572 w581 w590 w599 w608 w617 w626 w635 w644]
                    tunnel: w516 -> [w526 w535 w544 w553 w562 w571 w580 w589 w598 w607 w616 w625 w634 w643]
                    tunnel: [w525 w534 w543 w552 w561 w570 w579 w588 w597 w606 w615 w624 w633 w642] -> w515
                    tunnel: w514 -> [w523 w532 w541 w550 w559 w568 w577 w586 w595 w604 w613 w622 w631 w640]
                    tunnel: [w522 w531 w540 w549 w558 w566 w575 w584 w594 w603 w612 w621 w630 w639] -> w513
                    tunnel: w512 -> [w521 w530 w539 w548 w557 w567 w576 w585 w593 w602 w611 w620 w629 w638]
                    frame 0, Default {
                      n122 = call-poly <vilib>:"Read Key.vi"("section"=w527, "error in (no error)"=w526, "key"=w523, "refnum"=w529) -> ("error out"=w525:errorcluster, "value"=w524:string, "refnum out"=w528:T2)  [unwired: 4 in, 1 out]
                      n123 = Bundle By Name(cluster=w521, "規格"=w524) -> (w522:T1)
                    }
                    frame 1 {
                      n124 = call-poly <vilib>:"Read Key.vi"("section"=w536, "error in (no error)"=w535, "key"=w532, "refnum"=w538) -> ("error out"=w534:errorcluster, "value"=w533:string, "refnum out"=w537:T2)  [unwired: 4 in, 1 out]
                      n125 = Bundle By Name(cluster=w530, "規格上限"=w533) -> (w531:T1)
                    }
                    frame 2 {
                      n126 = call-poly <vilib>:"Read Key.vi"("section"=w545, "error in (no error)"=w544, "key"=w541, "refnum"=w547) -> ("error out"=w543:errorcluster, "value"=w542:string, "refnum out"=w546:T2)  [unwired: 4 in, 1 out]
                      n127 = Bundle By Name(cluster=w539, "規格下限"=w542) -> (w540:T1)
                    }
                    frame 3 {
                      n128 = call-poly <vilib>:"Read Key.vi"("section"=w554, "error in (no error)"=w553, "key"=w550, "refnum"=w556) -> ("error out"=w552:errorcluster, "value"=w551:i32, "refnum out"=w555:T2)  [unwired: 4 in, 1 out]
                      n129 = Bundle By Name(cluster=w548, "ポートNo."=w551) -> (w549:T1)
                    }
                    frame 4 {
                      n130 = call-poly <vilib>:"Read Key.vi"("section"=w563, "error in (no error)"=w562, "key"=w559, "refnum"=w565) -> ("error out"=w561:errorcluster, "value"=w560:i32, "refnum out"=w564:T2)  [unwired: 4 in, 1 out]
                      n131 = Bundle By Name(cluster=w557, "測定モード"=w560) -> (w558:T1)
                    }
                    frame 5 {
                      n132 = call-poly <vilib>:"Read Key.vi"("section"=w572, "error in (no error)"=w571, "key"=w568, "refnum"=w574) -> ("error out"=w570:errorcluster, "value"=w569:string, "refnum out"=w573:T2)  [unwired: 4 in, 1 out]
                      n133 = Bundle By Name(cluster=w567, "規格単位"=w569) -> (w566:T1)
                    }
                    frame 6 {
                      n134 = call-poly <vilib>:"Read Key.vi"("section"=w581, "error in (no error)"=w580, "key"=w577, "refnum"=w583) -> ("error out"=w579:errorcluster, "value"=w578:string, "refnum out"=w582:T2)  [unwired: 4 in, 1 out]
                      n135 = Bundle By Name(cluster=w576, "品質チェック項目"=w578) -> (w575:T1)
                    }
                    frame 7 {
                      n136 = call-poly <vilib>:"Read Key.vi"("section"=w590, "error in (no error)"=w589, "key"=w586, "refnum"=w592) -> ("error out"=w588:errorcluster, "value"=w587:i32, "refnum out"=w591:T2)  [unwired: 4 in, 1 out]
                      n137 = Bundle By Name(cluster=w585, "測定周期"=w587) -> (w584:T1)
                    }
                    frame 8 {
                      n138 = call-poly <vilib>:"Read Key.vi"("section"=w599, "error in (no error)"=w598, "key"=w595, "refnum"=w601) -> ("error out"=w597:errorcluster, "value"=w596:string, "refnum out"=w600:T2)  [unwired: 4 in, 1 out]
                      n139 = Bundle By Name(cluster=w593, "実測値MAX"=w596) -> (w594:T1)
                    }
                    frame 9 {
                      n140 = call-poly <vilib>:"Read Key.vi"("section"=w608, "error in (no error)"=w607, "key"=w604, "refnum"=w610) -> ("error out"=w606:errorcluster, "value"=w605:string, "refnum out"=w609:T2)  [unwired: 4 in, 1 out]
                      n141 = Bundle By Name(cluster=w602, "実測値MIN"=w605) -> (w603:T1)
                    }
                    frame 10 {
                      n142 = call-poly <vilib>:"Read Key.vi"("section"=w617, "error in (no error)"=w616, "key"=w613, "refnum"=w619) -> ("error out"=w615:errorcluster, "value"=w614:string, "refnum out"=w618:T2)  [unwired: 4 in, 1 out]
                      n143 = Bundle By Name(cluster=w611, "実測値(MAX)"=w614) -> (w612:T1)
                    }
                    frame 11 {
                      n144 = call-poly <vilib>:"Read Key.vi"("section"=w626, "error in (no error)"=w625, "key"=w622, "refnum"=w628) -> ("error out"=w624:errorcluster, "value"=w623:string, "refnum out"=w627:T2)  [unwired: 4 in, 1 out]
                      n145 = Bundle By Name(cluster=w620, "実測値(MIN)"=w623) -> (w621:T1)
                    }
                    frame 12 {
                      n146 = call-poly <vilib>:"Read Key.vi"("section"=w635, "error in (no error)"=w634, "key"=w631, "refnum"=w637) -> ("error out"=w633:errorcluster, "value"=w632:bool, "refnum out"=w636:T2)  [unwired: 4 in, 1 out]
                      n147 = Bundle By Name(cluster=w629, "測定画面表示ボタン"=w632) -> (w630:T1)
                    }
                    frame 13 {
                      n148 = call-poly <vilib>:"Read Key.vi"("section"=w644, "error in (no error)"=w643, "key"=w640, "refnum"=w646) -> ("error out"=w642:errorcluster, "value"=w641:string, "refnum out"=w645:T2)  [unwired: 4 in, 1 out]
                      n149 = Bundle By Name(cluster=w638, "ゲージポートNo"=w641) -> (w639:T1)
                    }
                  }
                  n150 = local write "メイン設定_設定 4"(w513) -> ()
                }
              }
              frame #1 {
                n151 = local read "メイン設定_設定 4"() -> (w647:T1)
              }
            }
            n152 = Replace Array Subset(array=w499, new element=w497, index=3) -> (w498:T1[])
          }
          frame 4 {
            # "③"
            n153 = flat-sequence {
              tunnel: w659 -> [w661]
              tunnel: w658 -> [w660]
              tunnel: [w665] -> w655
              tunnel: [w664] -> w654
              tunnel: [w802] -> w656
              tunnel: [w803] -> w657
              tunnel: w655 -> [w803]
              tunnel: w654 -> [w802]
              tunnel: [w801] -> w651
              frame #0 {
                # "④"
                # "setting.iniファイルからの設定項目の読み取り"
                n154 = for {
                  tunnel: "設定5" -> [w673]
                  tunnel: string[] ["規格", "規格上限", "規格下限", "ポートNo.", "測定モード", "規格単位", "品質チェック項目", "測定周期", "実測MAX", "実測MIN", "実測(MAX)", "実測(MIN)", "測定画面表示ボタン", "ゲージポートNo.", ""] -> [w668] mode=indexing
                  tunnel: w660 -> [w670]
                  tunnel: [w669] -> w664
                  tunnel: w661 -> [w674]
                  tunnel: [w672] -> w665
                  i -> [w671]
                  n155 = local read "メイン設定_設定 5"() -> (w666:T1)
                  n156 = case shown="1" w671 {
                    tunnel: w674 -> [w683 w692 w701 w710 w719 w728 w737 w746 w755 w764 w773 w782 w791 w800]
                    tunnel: [w682 w691 w700 w709 w718 w727 w736 w745 w754 w763 w772 w781 w790 w799] -> w672
                    tunnel: w673 -> [w681 w690 w699 w708 w717 w726 w735 w744 w753 w762 w771 w780 w789 w798]
                    tunnel: w670 -> [w680 w689 w698 w707 w716 w725 w734 w743 w752 w761 w770 w779 w788 w797]
                    tunnel: [w679 w688 w697 w706 w715 w724 w733 w742 w751 w760 w769 w778 w787 w796] -> w669
                    tunnel: w668 -> [w677 w686 w695 w704 w713 w722 w731 w740 w749 w758 w767 w776 w785 w794]
                    tunnel: [w676 w685 w694 w703 w712 w720 w729 w738 w748 w757 w766 w775 w784 w793] -> w667
                    tunnel: w666 -> [w675 w684 w693 w702 w711 w721 w730 w739 w747 w756 w765 w774 w783 w792]
                    frame 0, Default {
                      n157 = call-poly <vilib>:"Read Key.vi"("section"=w681, "error in (no error)"=w680, "key"=w677, "refnum"=w683) -> ("error out"=w679:errorcluster, "value"=w678:string, "refnum out"=w682:T2)  [unwired: 4 in, 1 out]
                      n158 = Bundle By Name(cluster=w675, "規格"=w678) -> (w676:T1)
                    }
                    frame 1 {
                      n159 = call-poly <vilib>:"Read Key.vi"("section"=w690, "error in (no error)"=w689, "key"=w686, "refnum"=w692) -> ("error out"=w688:errorcluster, "value"=w687:string, "refnum out"=w691:T2)  [unwired: 4 in, 1 out]
                      n160 = Bundle By Name(cluster=w684, "規格上限"=w687) -> (w685:T1)
                    }
                    frame 2 {
                      n161 = call-poly <vilib>:"Read Key.vi"("section"=w699, "error in (no error)"=w698, "key"=w695, "refnum"=w701) -> ("error out"=w697:errorcluster, "value"=w696:string, "refnum out"=w700:T2)  [unwired: 4 in, 1 out]
                      n162 = Bundle By Name(cluster=w693, "規格下限"=w696) -> (w694:T1)
                    }
                    frame 3 {
                      n163 = call-poly <vilib>:"Read Key.vi"("section"=w708, "error in (no error)"=w707, "key"=w704, "refnum"=w710) -> ("error out"=w706:errorcluster, "value"=w705:i32, "refnum out"=w709:T2)  [unwired: 4 in, 1 out]
                      n164 = Bundle By Name(cluster=w702, "ポートNo."=w705) -> (w703:T1)
                    }
                    frame 4 {
                      n165 = call-poly <vilib>:"Read Key.vi"("section"=w717, "error in (no error)"=w716, "key"=w713, "refnum"=w719) -> ("error out"=w715:errorcluster, "value"=w714:i32, "refnum out"=w718:T2)  [unwired: 4 in, 1 out]
                      n166 = Bundle By Name(cluster=w711, "測定モード"=w714) -> (w712:T1)
                    }
                    frame 5 {
                      n167 = call-poly <vilib>:"Read Key.vi"("section"=w726, "error in (no error)"=w725, "key"=w722, "refnum"=w728) -> ("error out"=w724:errorcluster, "value"=w723:string, "refnum out"=w727:T2)  [unwired: 4 in, 1 out]
                      n168 = Bundle By Name(cluster=w721, "規格単位"=w723) -> (w720:T1)
                    }
                    frame 6 {
                      n169 = call-poly <vilib>:"Read Key.vi"("section"=w735, "error in (no error)"=w734, "key"=w731, "refnum"=w737) -> ("error out"=w733:errorcluster, "value"=w732:string, "refnum out"=w736:T2)  [unwired: 4 in, 1 out]
                      n170 = Bundle By Name(cluster=w730, "品質チェック項目"=w732) -> (w729:T1)
                    }
                    frame 7 {
                      n171 = call-poly <vilib>:"Read Key.vi"("section"=w744, "error in (no error)"=w743, "key"=w740, "refnum"=w746) -> ("error out"=w742:errorcluster, "value"=w741:i32, "refnum out"=w745:T2)  [unwired: 4 in, 1 out]
                      n172 = Bundle By Name(cluster=w739, "測定周期"=w741) -> (w738:T1)
                    }
                    frame 8 {
                      n173 = call-poly <vilib>:"Read Key.vi"("section"=w753, "error in (no error)"=w752, "key"=w749, "refnum"=w755) -> ("error out"=w751:errorcluster, "value"=w750:string, "refnum out"=w754:T2)  [unwired: 4 in, 1 out]
                      n174 = Bundle By Name(cluster=w747, "実測値MAX"=w750) -> (w748:T1)
                    }
                    frame 9 {
                      n175 = call-poly <vilib>:"Read Key.vi"("section"=w762, "error in (no error)"=w761, "key"=w758, "refnum"=w764) -> ("error out"=w760:errorcluster, "value"=w759:string, "refnum out"=w763:T2)  [unwired: 4 in, 1 out]
                      n176 = Bundle By Name(cluster=w756, "実測値MIN"=w759) -> (w757:T1)
                    }
                    frame 10 {
                      n177 = call-poly <vilib>:"Read Key.vi"("section"=w771, "error in (no error)"=w770, "key"=w767, "refnum"=w773) -> ("error out"=w769:errorcluster, "value"=w768:string, "refnum out"=w772:T2)  [unwired: 4 in, 1 out]
                      n178 = Bundle By Name(cluster=w765, "実測値(MAX)"=w768) -> (w766:T1)
                    }
                    frame 11 {
                      n179 = call-poly <vilib>:"Read Key.vi"("section"=w780, "error in (no error)"=w779, "key"=w776, "refnum"=w782) -> ("error out"=w778:errorcluster, "value"=w777:string, "refnum out"=w781:T2)  [unwired: 4 in, 1 out]
                      n180 = Bundle By Name(cluster=w774, "実測値(MIN)"=w777) -> (w775:T1)
                    }
                    frame 12 {
                      n181 = call-poly <vilib>:"Read Key.vi"("section"=w789, "error in (no error)"=w788, "key"=w785, "refnum"=w791) -> ("error out"=w787:errorcluster, "value"=w786:bool, "refnum out"=w790:T2)  [unwired: 4 in, 1 out]
                      n182 = Bundle By Name(cluster=w783, "測定画面表示ボタン"=w786) -> (w784:T1)
                    }
                    frame 13 {
                      n183 = call-poly <vilib>:"Read Key.vi"("section"=w798, "error in (no error)"=w797, "key"=w794, "refnum"=w800) -> ("error out"=w796:errorcluster, "value"=w795:string, "refnum out"=w799:T2)  [unwired: 4 in, 1 out]
                      n184 = Bundle By Name(cluster=w792, "ゲージポートNo"=w795) -> (w793:T1)
                    }
                  }
                  n185 = local write "メイン設定_設定 5"(w667) -> ()
                }
              }
              frame #1 {
                n186 = local read "メイン設定_設定 5"() -> (w801:T1)
              }
            }
            n187 = Replace Array Subset(array=w653, new element=w651, index=4) -> (w652:T1[])
          }
          frame 5 {
            # "③"
            n188 = flat-sequence {
              tunnel: w813 -> [w815]
              tunnel: w812 -> [w814]
              tunnel: [w819] -> w809
              tunnel: [w818] -> w808
              tunnel: [w956] -> w810
              tunnel: [w957] -> w811
              tunnel: w809 -> [w957]
              tunnel: w808 -> [w956]
              tunnel: [w955] -> w805
              frame #0 {
                # "④"
                # "setting.iniファイルからの設定項目の読み取り"
                n189 = for {
                  tunnel: "設定6" -> [w827]
                  tunnel: string[] ["規格", "規格上限", "規格下限", "ポートNo.", "測定モード", "規格単位", "品質チェック項目", "測定周期", "実測MAX", "実測MIN", "実測(MAX)", "実測(MIN)", "測定画面表示ボタン", "ゲージポートNo.", ""] -> [w822] mode=indexing
                  tunnel: w814 -> [w824]
                  tunnel: [w823] -> w818
                  tunnel: w815 -> [w828]
                  tunnel: [w826] -> w819
                  i -> [w825]
                  n190 = local read "メイン設定_設定 6"() -> (w820:T1)
                  n191 = case shown="1" w825 {
                    tunnel: w828 -> [w837 w846 w855 w864 w873 w882 w891 w900 w909 w918 w927 w936 w945 w954]
                    tunnel: [w836 w845 w854 w863 w872 w881 w890 w899 w908 w917 w926 w935 w944 w953] -> w826
                    tunnel: w827 -> [w835 w844 w853 w862 w871 w880 w889 w898 w907 w916 w925 w934 w943 w952]
                    tunnel: w824 -> [w834 w843 w852 w861 w870 w879 w888 w897 w906 w915 w924 w933 w942 w951]
                    tunnel: [w833 w842 w851 w860 w869 w878 w887 w896 w905 w914 w923 w932 w941 w950] -> w823
                    tunnel: w822 -> [w831 w840 w849 w858 w867 w876 w885 w894 w903 w912 w921 w930 w939 w948]
                    tunnel: [w830 w839 w848 w857 w866 w874 w883 w892 w902 w911 w920 w929 w938 w947] -> w821
                    tunnel: w820 -> [w829 w838 w847 w856 w865 w875 w884 w893 w901 w910 w919 w928 w937 w946]
                    frame 0, Default {
                      n192 = call-poly <vilib>:"Read Key.vi"("section"=w835, "error in (no error)"=w834, "key"=w831, "refnum"=w837) -> ("error out"=w833:errorcluster, "value"=w832:string, "refnum out"=w836:T2)  [unwired: 4 in, 1 out]
                      n193 = Bundle By Name(cluster=w829, "規格"=w832) -> (w830:T1)
                    }
                    frame 1 {
                      n194 = call-poly <vilib>:"Read Key.vi"("section"=w844, "error in (no error)"=w843, "key"=w840, "refnum"=w846) -> ("error out"=w842:errorcluster, "value"=w841:string, "refnum out"=w845:T2)  [unwired: 4 in, 1 out]
                      n195 = Bundle By Name(cluster=w838, "規格上限"=w841) -> (w839:T1)
                    }
                    frame 2 {
                      n196 = call-poly <vilib>:"Read Key.vi"("section"=w853, "error in (no error)"=w852, "key"=w849, "refnum"=w855) -> ("error out"=w851:errorcluster, "value"=w850:string, "refnum out"=w854:T2)  [unwired: 4 in, 1 out]
                      n197 = Bundle By Name(cluster=w847, "規格下限"=w850) -> (w848:T1)
                    }
                    frame 3 {
                      n198 = call-poly <vilib>:"Read Key.vi"("section"=w862, "error in (no error)"=w861, "key"=w858, "refnum"=w864) -> ("error out"=w860:errorcluster, "value"=w859:i32, "refnum out"=w863:T2)  [unwired: 4 in, 1 out]
                      n199 = Bundle By Name(cluster=w856, "ポートNo."=w859) -> (w857:T1)
                    }
                    frame 4 {
                      n200 = call-poly <vilib>:"Read Key.vi"("section"=w871, "error in (no error)"=w870, "key"=w867, "refnum"=w873) -> ("error out"=w869:errorcluster, "value"=w868:i32, "refnum out"=w872:T2)  [unwired: 4 in, 1 out]
                      n201 = Bundle By Name(cluster=w865, "測定モード"=w868) -> (w866:T1)
                    }
                    frame 5 {
                      n202 = call-poly <vilib>:"Read Key.vi"("section"=w880, "error in (no error)"=w879, "key"=w876, "refnum"=w882) -> ("error out"=w878:errorcluster, "value"=w877:string, "refnum out"=w881:T2)  [unwired: 4 in, 1 out]
                      n203 = Bundle By Name(cluster=w875, "規格単位"=w877) -> (w874:T1)
                    }
                    frame 6 {
                      n204 = call-poly <vilib>:"Read Key.vi"("section"=w889, "error in (no error)"=w888, "key"=w885, "refnum"=w891) -> ("error out"=w887:errorcluster, "value"=w886:string, "refnum out"=w890:T2)  [unwired: 4 in, 1 out]
                      n205 = Bundle By Name(cluster=w884, "品質チェック項目"=w886) -> (w883:T1)
                    }
                    frame 7 {
                      n206 = call-poly <vilib>:"Read Key.vi"("section"=w898, "error in (no error)"=w897, "key"=w894, "refnum"=w900) -> ("error out"=w896:errorcluster, "value"=w895:i32, "refnum out"=w899:T2)  [unwired: 4 in, 1 out]
                      n207 = Bundle By Name(cluster=w893, "測定周期"=w895) -> (w892:T1)
                    }
                    frame 8 {
                      n208 = call-poly <vilib>:"Read Key.vi"("section"=w907, "error in (no error)"=w906, "key"=w903, "refnum"=w909) -> ("error out"=w905:errorcluster, "value"=w904:string, "refnum out"=w908:T2)  [unwired: 4 in, 1 out]
                      n209 = Bundle By Name(cluster=w901, "実測値MAX"=w904) -> (w902:T1)
                    }
                    frame 9 {
                      n210 = call-poly <vilib>:"Read Key.vi"("section"=w916, "error in (no error)"=w915, "key"=w912, "refnum"=w918) -> ("error out"=w914:errorcluster, "value"=w913:string, "refnum out"=w917:T2)  [unwired: 4 in, 1 out]
                      n211 = Bundle By Name(cluster=w910, "実測値MIN"=w913) -> (w911:T1)
                    }
                    frame 10 {
                      n212 = call-poly <vilib>:"Read Key.vi"("section"=w925, "error in (no error)"=w924, "key"=w921, "refnum"=w927) -> ("error out"=w923:errorcluster, "value"=w922:string, "refnum out"=w926:T2)  [unwired: 4 in, 1 out]
                      n213 = Bundle By Name(cluster=w919, "実測値(MAX)"=w922) -> (w920:T1)
                    }
                    frame 11 {
                      n214 = call-poly <vilib>:"Read Key.vi"("section"=w934, "error in (no error)"=w933, "key"=w930, "refnum"=w936) -> ("error out"=w932:errorcluster, "value"=w931:string, "refnum out"=w935:T2)  [unwired: 4 in, 1 out]
                      n215 = Bundle By Name(cluster=w928, "実測値(MIN)"=w931) -> (w929:T1)
                    }
                    frame 12 {
                      n216 = call-poly <vilib>:"Read Key.vi"("section"=w943, "error in (no error)"=w942, "key"=w939, "refnum"=w945) -> ("error out"=w941:errorcluster, "value"=w940:bool, "refnum out"=w944:T2)  [unwired: 4 in, 1 out]
                      n217 = Bundle By Name(cluster=w937, "測定画面表示ボタン"=w940) -> (w938:T1)
                    }
                    frame 13 {
                      n218 = call-poly <vilib>:"Read Key.vi"("section"=w952, "error in (no error)"=w951, "key"=w948, "refnum"=w954) -> ("error out"=w950:errorcluster, "value"=w949:string, "refnum out"=w953:T2)  [unwired: 4 in, 1 out]
                      n219 = Bundle By Name(cluster=w946, "ゲージポートNo"=w949) -> (w947:T1)
                    }
                  }
                  n220 = local write "メイン設定_設定 6"(w821) -> ()
                }
              }
              frame #1 {
                n221 = local read "メイン設定_設定 6"() -> (w955:T1)
              }
            }
            n222 = Replace Array Subset(array=w807, new element=w805, index=5) -> (w806:T1[])
          }
          frame 6 {
            # "③"
            n223 = flat-sequence {
              tunnel: w967 -> [w969]
              tunnel: w966 -> [w968]
              tunnel: [w973] -> w963
              tunnel: [w972] -> w962
              tunnel: [w1110] -> w964
              tunnel: [w1111] -> w965
              tunnel: w963 -> [w1111]
              tunnel: w962 -> [w1110]
              tunnel: [w1109] -> w959
              frame #0 {
                # "④"
                # "setting.iniファイルからの設定項目の読み取り"
                n224 = for {
                  tunnel: "設定7" -> [w981]
                  tunnel: string[] ["規格", "規格上限", "規格下限", "ポートNo.", "測定モード", "規格単位", "品質チェック項目", "測定周期", "実測MAX", "実測MIN", "実測(MAX)", "実測(MIN)", "測定画面表示ボタン", "ゲージポートNo.", ""] -> [w976] mode=indexing
                  tunnel: w968 -> [w978]
                  tunnel: [w977] -> w972
                  tunnel: w969 -> [w982]
                  tunnel: [w980] -> w973
                  i -> [w979]
                  n225 = local read "メイン設定_設定 7"() -> (w974:T1)
                  n226 = case shown="1" w979 {
                    tunnel: w982 -> [w991 w1000 w1009 w1018 w1027 w1036 w1045 w1054 w1063 w1072 w1081 w1090 w1099 w1108]
                    tunnel: [w990 w999 w1008 w1017 w1026 w1035 w1044 w1053 w1062 w1071 w1080 w1089 w1098 w1107] -> w980
                    tunnel: w981 -> [w989 w998 w1007 w1016 w1025 w1034 w1043 w1052 w1061 w1070 w1079 w1088 w1097 w1106]
                    tunnel: w978 -> [w988 w997 w1006 w1015 w1024 w1033 w1042 w1051 w1060 w1069 w1078 w1087 w1096 w1105]
                    tunnel: [w987 w996 w1005 w1014 w1023 w1032 w1041 w1050 w1059 w1068 w1077 w1086 w1095 w1104] -> w977
                    tunnel: w976 -> [w985 w994 w1003 w1012 w1021 w1030 w1039 w1048 w1057 w1066 w1075 w1084 w1093 w1102]
                    tunnel: [w984 w993 w1002 w1011 w1020 w1028 w1037 w1046 w1056 w1065 w1074 w1083 w1092 w1101] -> w975
                    tunnel: w974 -> [w983 w992 w1001 w1010 w1019 w1029 w1038 w1047 w1055 w1064 w1073 w1082 w1091 w1100]
                    frame 0, Default {
                      n227 = call-poly <vilib>:"Read Key.vi"("section"=w989, "error in (no error)"=w988, "key"=w985, "refnum"=w991) -> ("error out"=w987:errorcluster, "value"=w986:string, "refnum out"=w990:T2)  [unwired: 4 in, 1 out]
                      n228 = Bundle By Name(cluster=w983, "規格"=w986) -> (w984:T1)
                    }
                    frame 1 {
                      n229 = call-poly <vilib>:"Read Key.vi"("section"=w998, "error in (no error)"=w997, "key"=w994, "refnum"=w1000) -> ("error out"=w996:errorcluster, "value"=w995:string, "refnum out"=w999:T2)  [unwired: 4 in, 1 out]
                      n230 = Bundle By Name(cluster=w992, "規格上限"=w995) -> (w993:T1)
                    }
                    frame 2 {
                      n231 = call-poly <vilib>:"Read Key.vi"("section"=w1007, "error in (no error)"=w1006, "key"=w1003, "refnum"=w1009) -> ("error out"=w1005:errorcluster, "value"=w1004:string, "refnum out"=w1008:T2)  [unwired: 4 in, 1 out]
                      n232 = Bundle By Name(cluster=w1001, "規格下限"=w1004) -> (w1002:T1)
                    }
                    frame 3 {
                      n233 = call-poly <vilib>:"Read Key.vi"("section"=w1016, "error in (no error)"=w1015, "key"=w1012, "refnum"=w1018) -> ("error out"=w1014:errorcluster, "value"=w1013:i32, "refnum out"=w1017:T2)  [unwired: 4 in, 1 out]
                      n234 = Bundle By Name(cluster=w1010, "ポートNo."=w1013) -> (w1011:T1)
                    }
                    frame 4 {
                      n235 = call-poly <vilib>:"Read Key.vi"("section"=w1025, "error in (no error)"=w1024, "key"=w1021, "refnum"=w1027) -> ("error out"=w1023:errorcluster, "value"=w1022:i32, "refnum out"=w1026:T2)  [unwired: 4 in, 1 out]
                      n236 = Bundle By Name(cluster=w1019, "測定モード"=w1022) -> (w1020:T1)
                    }
                    frame 5 {
                      n237 = call-poly <vilib>:"Read Key.vi"("section"=w1034, "error in (no error)"=w1033, "key"=w1030, "refnum"=w1036) -> ("error out"=w1032:errorcluster, "value"=w1031:string, "refnum out"=w1035:T2)  [unwired: 4 in, 1 out]
                      n238 = Bundle By Name(cluster=w1029, "規格単位"=w1031) -> (w1028:T1)
                    }
                    frame 6 {
                      n239 = call-poly <vilib>:"Read Key.vi"("section"=w1043, "error in (no error)"=w1042, "key"=w1039, "refnum"=w1045) -> ("error out"=w1041:errorcluster, "value"=w1040:string, "refnum out"=w1044:T2)  [unwired: 4 in, 1 out]
                      n240 = Bundle By Name(cluster=w1038, "品質チェック項目"=w1040) -> (w1037:T1)
                    }
                    frame 7 {
                      n241 = call-poly <vilib>:"Read Key.vi"("section"=w1052, "error in (no error)"=w1051, "key"=w1048, "refnum"=w1054) -> ("error out"=w1050:errorcluster, "value"=w1049:i32, "refnum out"=w1053:T2)  [unwired: 4 in, 1 out]
                      n242 = Bundle By Name(cluster=w1047, "測定周期"=w1049) -> (w1046:T1)
                    }
                    frame 8 {
                      n243 = call-poly <vilib>:"Read Key.vi"("section"=w1061, "error in (no error)"=w1060, "key"=w1057, "refnum"=w1063) -> ("error out"=w1059:errorcluster, "value"=w1058:string, "refnum out"=w1062:T2)  [unwired: 4 in, 1 out]
                      n244 = Bundle By Name(cluster=w1055, "実測値MAX"=w1058) -> (w1056:T1)
                    }
                    frame 9 {
                      n245 = call-poly <vilib>:"Read Key.vi"("section"=w1070, "error in (no error)"=w1069, "key"=w1066, "refnum"=w1072) -> ("error out"=w1068:errorcluster, "value"=w1067:string, "refnum out"=w1071:T2)  [unwired: 4 in, 1 out]
                      n246 = Bundle By Name(cluster=w1064, "実測値MIN"=w1067) -> (w1065:T1)
                    }
                    frame 10 {
                      n247 = call-poly <vilib>:"Read Key.vi"("section"=w1079, "error in (no error)"=w1078, "key"=w1075, "refnum"=w1081) -> ("error out"=w1077:errorcluster, "value"=w1076:string, "refnum out"=w1080:T2)  [unwired: 4 in, 1 out]
                      n248 = Bundle By Name(cluster=w1073, "実測値(MAX)"=w1076) -> (w1074:T1)
                    }
                    frame 11 {
                      n249 = call-poly <vilib>:"Read Key.vi"("section"=w1088, "error in (no error)"=w1087, "key"=w1084, "refnum"=w1090) -> ("error out"=w1086:errorcluster, "value"=w1085:string, "refnum out"=w1089:T2)  [unwired: 4 in, 1 out]
                      n250 = Bundle By Name(cluster=w1082, "実測値(MIN)"=w1085) -> (w1083:T1)
                    }
                    frame 12 {
                      n251 = call-poly <vilib>:"Read Key.vi"("section"=w1097, "error in (no error)"=w1096, "key"=w1093, "refnum"=w1099) -> ("error out"=w1095:errorcluster, "value"=w1094:bool, "refnum out"=w1098:T2)  [unwired: 4 in, 1 out]
                      n252 = Bundle By Name(cluster=w1091, "測定画面表示ボタン"=w1094) -> (w1092:T1)
                    }
                    frame 13 {
                      n253 = call-poly <vilib>:"Read Key.vi"("section"=w1106, "error in (no error)"=w1105, "key"=w1102, "refnum"=w1108) -> ("error out"=w1104:errorcluster, "value"=w1103:string, "refnum out"=w1107:T2)  [unwired: 4 in, 1 out]
                      n254 = Bundle By Name(cluster=w1100, "ゲージポートNo"=w1103) -> (w1101:T1)
                    }
                  }
                  n255 = local write "メイン設定_設定 7"(w975) -> ()
                }
              }
              frame #1 {
                n256 = local read "メイン設定_設定 7"() -> (w1109:T1)
              }
            }
            n257 = Replace Array Subset(array=w961, new element=w959, index=6) -> (w960:T1[])
          }
          frame 7 {
            # "③"
            n258 = flat-sequence {
              tunnel: w1121 -> [w1123]
              tunnel: w1120 -> [w1122]
              tunnel: [w1127] -> w1117
              tunnel: [w1126] -> w1116
              tunnel: [w1264] -> w1118
              tunnel: [w1265] -> w1119
              tunnel: w1117 -> [w1265]
              tunnel: w1116 -> [w1264]
              tunnel: [w1263] -> w1113
              frame #0 {
                # "④"
                # "setting.iniファイルからの設定項目の読み取り"
                n259 = for {
                  tunnel: "設定8" -> [w1135]
                  tunnel: string[] ["規格", "規格上限", "規格下限", "ポートNo.", "測定モード", "規格単位", "品質チェック項目", "測定周期", "実測MAX", "実測MIN", "実測(MAX)", "実測(MIN)", "測定画面表示ボタン", "ゲージポートNo.", ""] -> [w1130] mode=indexing
                  tunnel: w1122 -> [w1132]
                  tunnel: [w1131] -> w1126
                  tunnel: w1123 -> [w1136]
                  tunnel: [w1134] -> w1127
                  i -> [w1133]
                  n260 = local read "メイン設定_設定 8"() -> (w1128:T1)
                  n261 = case shown="1" w1133 {
                    tunnel: w1136 -> [w1145 w1154 w1163 w1172 w1181 w1190 w1199 w1208 w1217 w1226 w1235 w1244 w1253 w1262]
                    tunnel: [w1144 w1153 w1162 w1171 w1180 w1189 w1198 w1207 w1216 w1225 w1234 w1243 w1252 w1261] -> w1134
                    tunnel: w1135 -> [w1143 w1152 w1161 w1170 w1179 w1188 w1197 w1206 w1215 w1224 w1233 w1242 w1251 w1260]
                    tunnel: w1132 -> [w1142 w1151 w1160 w1169 w1178 w1187 w1196 w1205 w1214 w1223 w1232 w1241 w1250 w1259]
                    tunnel: [w1141 w1150 w1159 w1168 w1177 w1186 w1195 w1204 w1213 w1222 w1231 w1240 w1249 w1258] -> w1131
                    tunnel: w1130 -> [w1139 w1148 w1157 w1166 w1175 w1184 w1193 w1202 w1211 w1220 w1229 w1238 w1247 w1256]
                    tunnel: [w1138 w1147 w1156 w1165 w1174 w1182 w1191 w1200 w1210 w1219 w1228 w1237 w1246 w1255] -> w1129
                    tunnel: w1128 -> [w1137 w1146 w1155 w1164 w1173 w1183 w1192 w1201 w1209 w1218 w1227 w1236 w1245 w1254]
                    frame 0, Default {
                      n262 = call-poly <vilib>:"Read Key.vi"("section"=w1143, "error in (no error)"=w1142, "key"=w1139, "refnum"=w1145) -> ("error out"=w1141:errorcluster, "value"=w1140:string, "refnum out"=w1144:T2)  [unwired: 4 in, 1 out]
                      n263 = Bundle By Name(cluster=w1137, "規格"=w1140) -> (w1138:T1)
                    }
                    frame 1 {
                      n264 = call-poly <vilib>:"Read Key.vi"("section"=w1152, "error in (no error)"=w1151, "key"=w1148, "refnum"=w1154) -> ("error out"=w1150:errorcluster, "value"=w1149:string, "refnum out"=w1153:T2)  [unwired: 4 in, 1 out]
                      n265 = Bundle By Name(cluster=w1146, "規格上限"=w1149) -> (w1147:T1)
                    }
                    frame 2 {
                      n266 = call-poly <vilib>:"Read Key.vi"("section"=w1161, "error in (no error)"=w1160, "key"=w1157, "refnum"=w1163) -> ("error out"=w1159:errorcluster, "value"=w1158:string, "refnum out"=w1162:T2)  [unwired: 4 in, 1 out]
                      n267 = Bundle By Name(cluster=w1155, "規格下限"=w1158) -> (w1156:T1)
                    }
                    frame 3 {
                      n268 = call-poly <vilib>:"Read Key.vi"("section"=w1170, "error in (no error)"=w1169, "key"=w1166, "refnum"=w1172) -> ("error out"=w1168:errorcluster, "value"=w1167:i32, "refnum out"=w1171:T2)  [unwired: 4 in, 1 out]
                      n269 = Bundle By Name(cluster=w1164, "ポートNo."=w1167) -> (w1165:T1)
                    }
                    frame 4 {
                      n270 = call-poly <vilib>:"Read Key.vi"("section"=w1179, "error in (no error)"=w1178, "key"=w1175, "refnum"=w1181) -> ("error out"=w1177:errorcluster, "value"=w1176:i32, "refnum out"=w1180:T2)  [unwired: 4 in, 1 out]
                      n271 = Bundle By Name(cluster=w1173, "測定モード"=w1176) -> (w1174:T1)
                    }
                    frame 5 {
                      n272 = call-poly <vilib>:"Read Key.vi"("section"=w1188, "error in (no error)"=w1187, "key"=w1184, "refnum"=w1190) -> ("error out"=w1186:errorcluster, "value"=w1185:string, "refnum out"=w1189:T2)  [unwired: 4 in, 1 out]
                      n273 = Bundle By Name(cluster=w1183, "規格単位"=w1185) -> (w1182:T1)
                    }
                    frame 6 {
                      n274 = call-poly <vilib>:"Read Key.vi"("section"=w1197, "error in (no error)"=w1196, "key"=w1193, "refnum"=w1199) -> ("error out"=w1195:errorcluster, "value"=w1194:string, "refnum out"=w1198:T2)  [unwired: 4 in, 1 out]
                      n275 = Bundle By Name(cluster=w1192, "品質チェック項目"=w1194) -> (w1191:T1)
                    }
                    frame 7 {
                      n276 = call-poly <vilib>:"Read Key.vi"("section"=w1206, "error in (no error)"=w1205, "key"=w1202, "refnum"=w1208) -> ("error out"=w1204:errorcluster, "value"=w1203:i32, "refnum out"=w1207:T2)  [unwired: 4 in, 1 out]
                      n277 = Bundle By Name(cluster=w1201, "測定周期"=w1203) -> (w1200:T1)
                    }
                    frame 8 {
                      n278 = call-poly <vilib>:"Read Key.vi"("section"=w1215, "error in (no error)"=w1214, "key"=w1211, "refnum"=w1217) -> ("error out"=w1213:errorcluster, "value"=w1212:string, "refnum out"=w1216:T2)  [unwired: 4 in, 1 out]
                      n279 = Bundle By Name(cluster=w1209, "実測値MAX"=w1212) -> (w1210:T1)
                    }
                    frame 9 {
                      n280 = call-poly <vilib>:"Read Key.vi"("section"=w1224, "error in (no error)"=w1223, "key"=w1220, "refnum"=w1226) -> ("error out"=w1222:errorcluster, "value"=w1221:string, "refnum out"=w1225:T2)  [unwired: 4 in, 1 out]
                      n281 = Bundle By Name(cluster=w1218, "実測値MIN"=w1221) -> (w1219:T1)
                    }
                    frame 10 {
                      n282 = call-poly <vilib>:"Read Key.vi"("section"=w1233, "error in (no error)"=w1232, "key"=w1229, "refnum"=w1235) -> ("error out"=w1231:errorcluster, "value"=w1230:string, "refnum out"=w1234:T2)  [unwired: 4 in, 1 out]
                      n283 = Bundle By Name(cluster=w1227, "実測値(MAX)"=w1230) -> (w1228:T1)
                    }
                    frame 11 {
                      n284 = call-poly <vilib>:"Read Key.vi"("section"=w1242, "error in (no error)"=w1241, "key"=w1238, "refnum"=w1244) -> ("error out"=w1240:errorcluster, "value"=w1239:string, "refnum out"=w1243:T2)  [unwired: 4 in, 1 out]
                      n285 = Bundle By Name(cluster=w1236, "実測値(MIN)"=w1239) -> (w1237:T1)
                    }
                    frame 12 {
                      n286 = call-poly <vilib>:"Read Key.vi"("section"=w1251, "error in (no error)"=w1250, "key"=w1247, "refnum"=w1253) -> ("error out"=w1249:errorcluster, "value"=w1248:bool, "refnum out"=w1252:T2)  [unwired: 4 in, 1 out]
                      n287 = Bundle By Name(cluster=w1245, "測定画面表示ボタン"=w1248) -> (w1246:T1)
                    }
                    frame 13 {
                      n288 = call-poly <vilib>:"Read Key.vi"("section"=w1260, "error in (no error)"=w1259, "key"=w1256, "refnum"=w1262) -> ("error out"=w1258:errorcluster, "value"=w1257:string, "refnum out"=w1261:T2)  [unwired: 4 in, 1 out]
                      n289 = Bundle By Name(cluster=w1254, "ゲージポートNo"=w1257) -> (w1255:T1)
                    }
                  }
                  n290 = local write "メイン設定_設定 8"(w1129) -> ()
                }
              }
              frame #1 {
                n291 = local read "メイン設定_設定 8"() -> (w1263:T1)
              }
            }
            n292 = Replace Array Subset(array=w1115, new element=w1113, index=7) -> (w1114:T1[])
          }
          frame 8 {
            # "③"
            n293 = flat-sequence {
              tunnel: w1275 -> [w1277]
              tunnel: w1274 -> [w1276]
              tunnel: [w1281] -> w1271
              tunnel: [w1280] -> w1270
              tunnel: [w1418] -> w1272
              tunnel: [w1419] -> w1273
              tunnel: w1271 -> [w1419]
              tunnel: w1270 -> [w1418]
              tunnel: [w1417] -> w1267
              frame #0 {
                # "④"
                # "setting.iniファイルからの設定項目の読み取り"
                n294 = for {
                  tunnel: "設定9" -> [w1289]
                  tunnel: string[] ["規格", "規格上限", "規格下限", "ポートNo.", "測定モード", "規格単位", "品質チェック項目", "測定周期", "実測MAX", "実測MIN", "実測(MAX)", "実測(MIN)", "測定画面表示ボタン", "ゲージポートNo.", ""] -> [w1284] mode=indexing
                  tunnel: w1276 -> [w1286]
                  tunnel: [w1285] -> w1280
                  tunnel: w1277 -> [w1290]
                  tunnel: [w1288] -> w1281
                  i -> [w1287]
                  n295 = local read "メイン設定_設定 9"() -> (w1282:T1)
                  n296 = case shown="1" w1287 {
                    tunnel: w1290 -> [w1299 w1308 w1317 w1326 w1335 w1344 w1353 w1362 w1371 w1380 w1389 w1398 w1407 w1416]
                    tunnel: [w1298 w1307 w1316 w1325 w1334 w1343 w1352 w1361 w1370 w1379 w1388 w1397 w1406 w1415] -> w1288
                    tunnel: w1289 -> [w1297 w1306 w1315 w1324 w1333 w1342 w1351 w1360 w1369 w1378 w1387 w1396 w1405 w1414]
                    tunnel: w1286 -> [w1296 w1305 w1314 w1323 w1332 w1341 w1350 w1359 w1368 w1377 w1386 w1395 w1404 w1413]
                    tunnel: [w1295 w1304 w1313 w1322 w1331 w1340 w1349 w1358 w1367 w1376 w1385 w1394 w1403 w1412] -> w1285
                    tunnel: w1284 -> [w1293 w1302 w1311 w1320 w1329 w1338 w1347 w1356 w1365 w1374 w1383 w1392 w1401 w1410]
                    tunnel: [w1292 w1301 w1310 w1319 w1328 w1336 w1345 w1354 w1364 w1373 w1382 w1391 w1400 w1409] -> w1283
                    tunnel: w1282 -> [w1291 w1300 w1309 w1318 w1327 w1337 w1346 w1355 w1363 w1372 w1381 w1390 w1399 w1408]
                    frame 0, Default {
                      n297 = call-poly <vilib>:"Read Key.vi"("section"=w1297, "error in (no error)"=w1296, "key"=w1293, "refnum"=w1299) -> ("error out"=w1295:errorcluster, "value"=w1294:string, "refnum out"=w1298:T2)  [unwired: 4 in, 1 out]
                      n298 = Bundle By Name(cluster=w1291, "規格"=w1294) -> (w1292:T1)
                    }
                    frame 1 {
                      n299 = call-poly <vilib>:"Read Key.vi"("section"=w1306, "error in (no error)"=w1305, "key"=w1302, "refnum"=w1308) -> ("error out"=w1304:errorcluster, "value"=w1303:string, "refnum out"=w1307:T2)  [unwired: 4 in, 1 out]
                      n300 = Bundle By Name(cluster=w1300, "規格上限"=w1303) -> (w1301:T1)
                    }
                    frame 2 {
                      n301 = call-poly <vilib>:"Read Key.vi"("section"=w1315, "error in (no error)"=w1314, "key"=w1311, "refnum"=w1317) -> ("error out"=w1313:errorcluster, "value"=w1312:string, "refnum out"=w1316:T2)  [unwired: 4 in, 1 out]
                      n302 = Bundle By Name(cluster=w1309, "規格下限"=w1312) -> (w1310:T1)
                    }
                    frame 3 {
                      n303 = call-poly <vilib>:"Read Key.vi"("section"=w1324, "error in (no error)"=w1323, "key"=w1320, "refnum"=w1326) -> ("error out"=w1322:errorcluster, "value"=w1321:i32, "refnum out"=w1325:T2)  [unwired: 4 in, 1 out]
                      n304 = Bundle By Name(cluster=w1318, "ポートNo."=w1321) -> (w1319:T1)
                    }
                    frame 4 {
                      n305 = call-poly <vilib>:"Read Key.vi"("section"=w1333, "error in (no error)"=w1332, "key"=w1329, "refnum"=w1335) -> ("error out"=w1331:errorcluster, "value"=w1330:i32, "refnum out"=w1334:T2)  [unwired: 4 in, 1 out]
                      n306 = Bundle By Name(cluster=w1327, "測定モード"=w1330) -> (w1328:T1)
                    }
                    frame 5 {
                      n307 = call-poly <vilib>:"Read Key.vi"("section"=w1342, "error in (no error)"=w1341, "key"=w1338, "refnum"=w1344) -> ("error out"=w1340:errorcluster, "value"=w1339:string, "refnum out"=w1343:T2)  [unwired: 4 in, 1 out]
                      n308 = Bundle By Name(cluster=w1337, "規格単位"=w1339) -> (w1336:T1)
                    }
                    frame 6 {
                      n309 = call-poly <vilib>:"Read Key.vi"("section"=w1351, "error in (no error)"=w1350, "key"=w1347, "refnum"=w1353) -> ("error out"=w1349:errorcluster, "value"=w1348:string, "refnum out"=w1352:T2)  [unwired: 4 in, 1 out]
                      n310 = Bundle By Name(cluster=w1346, "品質チェック項目"=w1348) -> (w1345:T1)
                    }
                    frame 7 {
                      n311 = call-poly <vilib>:"Read Key.vi"("section"=w1360, "error in (no error)"=w1359, "key"=w1356, "refnum"=w1362) -> ("error out"=w1358:errorcluster, "value"=w1357:i32, "refnum out"=w1361:T2)  [unwired: 4 in, 1 out]
                      n312 = Bundle By Name(cluster=w1355, "測定周期"=w1357) -> (w1354:T1)
                    }
                    frame 8 {
                      n313 = call-poly <vilib>:"Read Key.vi"("section"=w1369, "error in (no error)"=w1368, "key"=w1365, "refnum"=w1371) -> ("error out"=w1367:errorcluster, "value"=w1366:string, "refnum out"=w1370:T2)  [unwired: 4 in, 1 out]
                      n314 = Bundle By Name(cluster=w1363, "実測値MAX"=w1366) -> (w1364:T1)
                    }
                    frame 9 {
                      n315 = call-poly <vilib>:"Read Key.vi"("section"=w1378, "error in (no error)"=w1377, "key"=w1374, "refnum"=w1380) -> ("error out"=w1376:errorcluster, "value"=w1375:string, "refnum out"=w1379:T2)  [unwired: 4 in, 1 out]
                      n316 = Bundle By Name(cluster=w1372, "実測値MIN"=w1375) -> (w1373:T1)
                    }
                    frame 10 {
                      n317 = call-poly <vilib>:"Read Key.vi"("section"=w1387, "error in (no error)"=w1386, "key"=w1383, "refnum"=w1389) -> ("error out"=w1385:errorcluster, "value"=w1384:string, "refnum out"=w1388:T2)  [unwired: 4 in, 1 out]
                      n318 = Bundle By Name(cluster=w1381, "実測値(MAX)"=w1384) -> (w1382:T1)
                    }
                    frame 11 {
                      n319 = call-poly <vilib>:"Read Key.vi"("section"=w1396, "error in (no error)"=w1395, "key"=w1392, "refnum"=w1398) -> ("error out"=w1394:errorcluster, "value"=w1393:string, "refnum out"=w1397:T2)  [unwired: 4 in, 1 out]
                      n320 = Bundle By Name(cluster=w1390, "実測値(MIN)"=w1393) -> (w1391:T1)
                    }
                    frame 12 {
                      n321 = call-poly <vilib>:"Read Key.vi"("section"=w1405, "error in (no error)"=w1404, "key"=w1401, "refnum"=w1407) -> ("error out"=w1403:errorcluster, "value"=w1402:bool, "refnum out"=w1406:T2)  [unwired: 4 in, 1 out]
                      n322 = Bundle By Name(cluster=w1399, "測定画面表示ボタン"=w1402) -> (w1400:T1)
                    }
                    frame 13 {
                      n323 = call-poly <vilib>:"Read Key.vi"("section"=w1414, "error in (no error)"=w1413, "key"=w1410, "refnum"=w1416) -> ("error out"=w1412:errorcluster, "value"=w1411:string, "refnum out"=w1415:T2)  [unwired: 4 in, 1 out]
                      n324 = Bundle By Name(cluster=w1408, "ゲージポートNo"=w1411) -> (w1409:T1)
                    }
                  }
                  n325 = local write "メイン設定_設定 9"(w1283) -> ()
                }
              }
              frame #1 {
                n326 = local read "メイン設定_設定 9"() -> (w1417:T1)
              }
            }
            n327 = Replace Array Subset(array=w1269, new element=w1267, index=8) -> (w1268:T1[])
          }
          frame 9 {
            # "③"
            n328 = flat-sequence {
              tunnel: w1429 -> [w1431]
              tunnel: w1428 -> [w1430]
              tunnel: [w1435] -> w1425
              tunnel: [w1434] -> w1424
              tunnel: [w1572] -> w1426
              tunnel: [w1573] -> w1427
              tunnel: w1425 -> [w1573]
              tunnel: w1424 -> [w1572]
              tunnel: [w1571] -> w1421
              frame #0 {
                # "④"
                # "setting.iniファイルからの設定項目の読み取り"
                n329 = for {
                  tunnel: "設定10" -> [w1443]
                  tunnel: string[] ["規格", "規格上限", "規格下限", "ポートNo.", "測定モード", "規格単位", "品質チェック項目", "測定周期", "実測MAX", "実測MIN", "実測(MAX)", "実測(MIN)", "測定画面表示ボタン", "ゲージポートNo.", ""] -> [w1438] mode=indexing
                  tunnel: w1430 -> [w1440]
                  tunnel: [w1439] -> w1434
                  tunnel: w1431 -> [w1444]
                  tunnel: [w1442] -> w1435
                  i -> [w1441]
                  n330 = local read "メイン設定_設定 10"() -> (w1436:T1)
                  n331 = case shown="1" w1441 {
                    tunnel: w1444 -> [w1453 w1462 w1471 w1480 w1489 w1498 w1507 w1516 w1525 w1534 w1543 w1552 w1561 w1570]
                    tunnel: [w1452 w1461 w1470 w1479 w1488 w1497 w1506 w1515 w1524 w1533 w1542 w1551 w1560 w1569] -> w1442
                    tunnel: w1443 -> [w1451 w1460 w1469 w1478 w1487 w1496 w1505 w1514 w1523 w1532 w1541 w1550 w1559 w1568]
                    tunnel: w1440 -> [w1450 w1459 w1468 w1477 w1486 w1495 w1504 w1513 w1522 w1531 w1540 w1549 w1558 w1567]
                    tunnel: [w1449 w1458 w1467 w1476 w1485 w1494 w1503 w1512 w1521 w1530 w1539 w1548 w1557 w1566] -> w1439
                    tunnel: w1438 -> [w1447 w1456 w1465 w1474 w1483 w1492 w1501 w1510 w1519 w1528 w1537 w1546 w1555 w1564]
                    tunnel: [w1446 w1455 w1464 w1473 w1482 w1490 w1499 w1508 w1518 w1527 w1536 w1545 w1554 w1563] -> w1437
                    tunnel: w1436 -> [w1445 w1454 w1463 w1472 w1481 w1491 w1500 w1509 w1517 w1526 w1535 w1544 w1553 w1562]
                    frame 0, Default {
                      n332 = call-poly <vilib>:"Read Key.vi"("section"=w1451, "error in (no error)"=w1450, "key"=w1447, "refnum"=w1453) -> ("error out"=w1449:errorcluster, "value"=w1448:string, "refnum out"=w1452:T2)  [unwired: 4 in, 1 out]
                      n333 = Bundle By Name(cluster=w1445, "規格"=w1448) -> (w1446:T1)
                    }
                    frame 1 {
                      n334 = call-poly <vilib>:"Read Key.vi"("section"=w1460, "error in (no error)"=w1459, "key"=w1456, "refnum"=w1462) -> ("error out"=w1458:errorcluster, "value"=w1457:string, "refnum out"=w1461:T2)  [unwired: 4 in, 1 out]
                      n335 = Bundle By Name(cluster=w1454, "規格上限"=w1457) -> (w1455:T1)
                    }
                    frame 2 {
                      n336 = call-poly <vilib>:"Read Key.vi"("section"=w1469, "error in (no error)"=w1468, "key"=w1465, "refnum"=w1471) -> ("error out"=w1467:errorcluster, "value"=w1466:string, "refnum out"=w1470:T2)  [unwired: 4 in, 1 out]
                      n337 = Bundle By Name(cluster=w1463, "規格下限"=w1466) -> (w1464:T1)
                    }
                    frame 3 {
                      n338 = call-poly <vilib>:"Read Key.vi"("section"=w1478, "error in (no error)"=w1477, "key"=w1474, "refnum"=w1480) -> ("error out"=w1476:errorcluster, "value"=w1475:i32, "refnum out"=w1479:T2)  [unwired: 4 in, 1 out]
                      n339 = Bundle By Name(cluster=w1472, "ポートNo."=w1475) -> (w1473:T1)
                    }
                    frame 4 {
                      n340 = call-poly <vilib>:"Read Key.vi"("section"=w1487, "error in (no error)"=w1486, "key"=w1483, "refnum"=w1489) -> ("error out"=w1485:errorcluster, "value"=w1484:i32, "refnum out"=w1488:T2)  [unwired: 4 in, 1 out]
                      n341 = Bundle By Name(cluster=w1481, "測定モード"=w1484) -> (w1482:T1)
                    }
                    frame 5 {
                      n342 = call-poly <vilib>:"Read Key.vi"("section"=w1496, "error in (no error)"=w1495, "key"=w1492, "refnum"=w1498) -> ("error out"=w1494:errorcluster, "value"=w1493:string, "refnum out"=w1497:T2)  [unwired: 4 in, 1 out]
                      n343 = Bundle By Name(cluster=w1491, "規格単位"=w1493) -> (w1490:T1)
                    }
                    frame 6 {
                      n344 = call-poly <vilib>:"Read Key.vi"("section"=w1505, "error in (no error)"=w1504, "key"=w1501, "refnum"=w1507) -> ("error out"=w1503:errorcluster, "value"=w1502:string, "refnum out"=w1506:T2)  [unwired: 4 in, 1 out]
                      n345 = Bundle By Name(cluster=w1500, "品質チェック項目"=w1502) -> (w1499:T1)
                    }
                    frame 7 {
                      n346 = call-poly <vilib>:"Read Key.vi"("section"=w1514, "error in (no error)"=w1513, "key"=w1510, "refnum"=w1516) -> ("error out"=w1512:errorcluster, "value"=w1511:i32, "refnum out"=w1515:T2)  [unwired: 4 in, 1 out]
                      n347 = Bundle By Name(cluster=w1509, "測定周期"=w1511) -> (w1508:T1)
                    }
                    frame 8 {
                      n348 = call-poly <vilib>:"Read Key.vi"("section"=w1523, "error in (no error)"=w1522, "key"=w1519, "refnum"=w1525) -> ("error out"=w1521:errorcluster, "value"=w1520:string, "refnum out"=w1524:T2)  [unwired: 4 in, 1 out]
                      n349 = Bundle By Name(cluster=w1517, "実測値MAX"=w1520) -> (w1518:T1)
                    }
                    frame 9 {
                      n350 = call-poly <vilib>:"Read Key.vi"("section"=w1532, "error in (no error)"=w1531, "key"=w1528, "refnum"=w1534) -> ("error out"=w1530:errorcluster, "value"=w1529:string, "refnum out"=w1533:T2)  [unwired: 4 in, 1 out]
                      n351 = Bundle By Name(cluster=w1526, "実測値MIN"=w1529) -> (w1527:T1)
                    }
                    frame 10 {
                      n352 = call-poly <vilib>:"Read Key.vi"("section"=w1541, "error in (no error)"=w1540, "key"=w1537, "refnum"=w1543) -> ("error out"=w1539:errorcluster, "value"=w1538:string, "refnum out"=w1542:T2)  [unwired: 4 in, 1 out]
                      n353 = Bundle By Name(cluster=w1535, "実測値(MAX)"=w1538) -> (w1536:T1)
                    }
                    frame 11 {
                      n354 = call-poly <vilib>:"Read Key.vi"("section"=w1550, "error in (no error)"=w1549, "key"=w1546, "refnum"=w1552) -> ("error out"=w1548:errorcluster, "value"=w1547:string, "refnum out"=w1551:T2)  [unwired: 4 in, 1 out]
                      n355 = Bundle By Name(cluster=w1544, "実測値(MIN)"=w1547) -> (w1545:T1)
                    }
                    frame 12 {
                      n356 = call-poly <vilib>:"Read Key.vi"("section"=w1559, "error in (no error)"=w1558, "key"=w1555, "refnum"=w1561) -> ("error out"=w1557:errorcluster, "value"=w1556:bool, "refnum out"=w1560:T2)  [unwired: 4 in, 1 out]
                      n357 = Bundle By Name(cluster=w1553, "測定画面表示ボタン"=w1556) -> (w1554:T1)
                    }
                    frame 13 {
                      n358 = call-poly <vilib>:"Read Key.vi"("section"=w1568, "error in (no error)"=w1567, "key"=w1564, "refnum"=w1570) -> ("error out"=w1566:errorcluster, "value"=w1565:string, "refnum out"=w1569:T2)  [unwired: 4 in, 1 out]
                      n359 = Bundle By Name(cluster=w1562, "ゲージポートNo"=w1565) -> (w1563:T1)
                    }
                  }
                  n360 = local write "メイン設定_設定 10"(w1437) -> ()
                }
              }
              frame #1 {
                n361 = local read "メイン設定_設定 10"() -> (w1571:T1)
              }
            }
            n362 = Replace Array Subset(array=w1423, new element=w1421, index=9) -> (w1422:T1[])
          }
          frame 10 {
            # "③"
            n363 = flat-sequence {
              tunnel: w1583 -> [w1585]
              tunnel: w1582 -> [w1584]
              tunnel: [w1589] -> w1579
              tunnel: [w1588] -> w1578
              tunnel: [w1726] -> w1580
              tunnel: [w1727] -> w1581
              tunnel: w1579 -> [w1727]
              tunnel: w1578 -> [w1726]
              tunnel: [w1725] -> w1575
              frame #0 {
                # "④"
                # "setting.iniファイルからの設定項目の読み取り"
                n364 = for {
                  tunnel: "設定11" -> [w1597]
                  tunnel: string[] ["規格", "規格上限", "規格下限", "ポートNo.", "測定モード", "規格単位", "品質チェック項目", "測定周期", "実測MAX", "実測MIN", "実測(MAX)", "実測(MIN)", "測定画面表示ボタン", "ゲージポートNo.", ""] -> [w1592] mode=indexing
                  tunnel: w1584 -> [w1594]
                  tunnel: [w1593] -> w1588
                  tunnel: w1585 -> [w1598]
                  tunnel: [w1596] -> w1589
                  i -> [w1595]
                  n365 = local read "メイン設定_設定 11"() -> (w1590:T1)
                  n366 = case shown="1" w1595 {
                    tunnel: w1598 -> [w1607 w1616 w1625 w1634 w1643 w1652 w1661 w1670 w1679 w1688 w1697 w1706 w1715 w1724]
                    tunnel: [w1606 w1615 w1624 w1633 w1642 w1651 w1660 w1669 w1678 w1687 w1696 w1705 w1714 w1723] -> w1596
                    tunnel: w1597 -> [w1605 w1614 w1623 w1632 w1641 w1650 w1659 w1668 w1677 w1686 w1695 w1704 w1713 w1722]
                    tunnel: w1594 -> [w1604 w1613 w1622 w1631 w1640 w1649 w1658 w1667 w1676 w1685 w1694 w1703 w1712 w1721]
                    tunnel: [w1603 w1612 w1621 w1630 w1639 w1648 w1657 w1666 w1675 w1684 w1693 w1702 w1711 w1720] -> w1593
                    tunnel: w1592 -> [w1601 w1610 w1619 w1628 w1637 w1646 w1655 w1664 w1673 w1682 w1691 w1700 w1709 w1718]
                    tunnel: [w1600 w1609 w1618 w1627 w1636 w1644 w1653 w1662 w1672 w1681 w1690 w1699 w1708 w1717] -> w1591
                    tunnel: w1590 -> [w1599 w1608 w1617 w1626 w1635 w1645 w1654 w1663 w1671 w1680 w1689 w1698 w1707 w1716]
                    frame 0, Default {
                      n367 = call-poly <vilib>:"Read Key.vi"("section"=w1605, "error in (no error)"=w1604, "key"=w1601, "refnum"=w1607) -> ("error out"=w1603:errorcluster, "value"=w1602:string, "refnum out"=w1606:T2)  [unwired: 4 in, 1 out]
                      n368 = Bundle By Name(cluster=w1599, "規格"=w1602) -> (w1600:T1)
                    }
                    frame 1 {
                      n369 = call-poly <vilib>:"Read Key.vi"("section"=w1614, "error in (no error)"=w1613, "key"=w1610, "refnum"=w1616) -> ("error out"=w1612:errorcluster, "value"=w1611:string, "refnum out"=w1615:T2)  [unwired: 4 in, 1 out]
                      n370 = Bundle By Name(cluster=w1608, "規格上限"=w1611) -> (w1609:T1)
                    }
                    frame 2 {
                      n371 = call-poly <vilib>:"Read Key.vi"("section"=w1623, "error in (no error)"=w1622, "key"=w1619, "refnum"=w1625) -> ("error out"=w1621:errorcluster, "value"=w1620:string, "refnum out"=w1624:T2)  [unwired: 4 in, 1 out]
                      n372 = Bundle By Name(cluster=w1617, "規格下限"=w1620) -> (w1618:T1)
                    }
                    frame 3 {
                      n373 = call-poly <vilib>:"Read Key.vi"("section"=w1632, "error in (no error)"=w1631, "key"=w1628, "refnum"=w1634) -> ("error out"=w1630:errorcluster, "value"=w1629:i32, "refnum out"=w1633:T2)  [unwired: 4 in, 1 out]
                      n374 = Bundle By Name(cluster=w1626, "ポートNo."=w1629) -> (w1627:T1)
                    }
                    frame 4 {
                      n375 = call-poly <vilib>:"Read Key.vi"("section"=w1641, "error in (no error)"=w1640, "key"=w1637, "refnum"=w1643) -> ("error out"=w1639:errorcluster, "value"=w1638:i32, "refnum out"=w1642:T2)  [unwired: 4 in, 1 out]
                      n376 = Bundle By Name(cluster=w1635, "測定モード"=w1638) -> (w1636:T1)
                    }
                    frame 5 {
                      n377 = call-poly <vilib>:"Read Key.vi"("section"=w1650, "error in (no error)"=w1649, "key"=w1646, "refnum"=w1652) -> ("error out"=w1648:errorcluster, "value"=w1647:string, "refnum out"=w1651:T2)  [unwired: 4 in, 1 out]
                      n378 = Bundle By Name(cluster=w1645, "規格単位"=w1647) -> (w1644:T1)
                    }
                    frame 6 {
                      n379 = call-poly <vilib>:"Read Key.vi"("section"=w1659, "error in (no error)"=w1658, "key"=w1655, "refnum"=w1661) -> ("error out"=w1657:errorcluster, "value"=w1656:string, "refnum out"=w1660:T2)  [unwired: 4 in, 1 out]
                      n380 = Bundle By Name(cluster=w1654, "品質チェック項目"=w1656) -> (w1653:T1)
                    }
                    frame 7 {
                      n381 = call-poly <vilib>:"Read Key.vi"("section"=w1668, "error in (no error)"=w1667, "key"=w1664, "refnum"=w1670) -> ("error out"=w1666:errorcluster, "value"=w1665:i32, "refnum out"=w1669:T2)  [unwired: 4 in, 1 out]
                      n382 = Bundle By Name(cluster=w1663, "測定周期"=w1665) -> (w1662:T1)
                    }
                    frame 8 {
                      n383 = call-poly <vilib>:"Read Key.vi"("section"=w1677, "error in (no error)"=w1676, "key"=w1673, "refnum"=w1679) -> ("error out"=w1675:errorcluster, "value"=w1674:string, "refnum out"=w1678:T2)  [unwired: 4 in, 1 out]
                      n384 = Bundle By Name(cluster=w1671, "実測値MAX"=w1674) -> (w1672:T1)
                    }
                    frame 9 {
                      n385 = call-poly <vilib>:"Read Key.vi"("section"=w1686, "error in (no error)"=w1685, "key"=w1682, "refnum"=w1688) -> ("error out"=w1684:errorcluster, "value"=w1683:string, "refnum out"=w1687:T2)  [unwired: 4 in, 1 out]
                      n386 = Bundle By Name(cluster=w1680, "実測値MIN"=w1683) -> (w1681:T1)
                    }
                    frame 10 {
                      n387 = call-poly <vilib>:"Read Key.vi"("section"=w1695, "error in (no error)"=w1694, "key"=w1691, "refnum"=w1697) -> ("error out"=w1693:errorcluster, "value"=w1692:string, "refnum out"=w1696:T2)  [unwired: 4 in, 1 out]
                      n388 = Bundle By Name(cluster=w1689, "実測値(MAX)"=w1692) -> (w1690:T1)
                    }
                    frame 11 {
                      n389 = call-poly <vilib>:"Read Key.vi"("section"=w1704, "error in (no error)"=w1703, "key"=w1700, "refnum"=w1706) -> ("error out"=w1702:errorcluster, "value"=w1701:string, "refnum out"=w1705:T2)  [unwired: 4 in, 1 out]
                      n390 = Bundle By Name(cluster=w1698, "実測値(MIN)"=w1701) -> (w1699:T1)
                    }
                    frame 12 {
                      n391 = call-poly <vilib>:"Read Key.vi"("section"=w1713, "error in (no error)"=w1712, "key"=w1709, "refnum"=w1715) -> ("error out"=w1711:errorcluster, "value"=w1710:bool, "refnum out"=w1714:T2)  [unwired: 4 in, 1 out]
                      n392 = Bundle By Name(cluster=w1707, "測定画面表示ボタン"=w1710) -> (w1708:T1)
                    }
                    frame 13 {
                      n393 = call-poly <vilib>:"Read Key.vi"("section"=w1722, "error in (no error)"=w1721, "key"=w1718, "refnum"=w1724) -> ("error out"=w1720:errorcluster, "value"=w1719:string, "refnum out"=w1723:T2)  [unwired: 4 in, 1 out]
                      n394 = Bundle By Name(cluster=w1716, "ゲージポートNo"=w1719) -> (w1717:T1)
                    }
                  }
                  n395 = local write "メイン設定_設定 11"(w1591) -> ()
                }
              }
              frame #1 {
                n396 = local read "メイン設定_設定 11"() -> (w1725:T1)
              }
            }
            n397 = Replace Array Subset(array=w1577, new element=w1575, index=10) -> (w1576:T1[])
          }
          frame 11 {
            # "③"
            n398 = flat-sequence {
              tunnel: w1737 -> [w1739]
              tunnel: w1736 -> [w1738]
              tunnel: [w1743] -> w1733
              tunnel: [w1742] -> w1732
              tunnel: [w1880] -> w1734
              tunnel: [w1881] -> w1735
              tunnel: w1733 -> [w1881]
              tunnel: w1732 -> [w1880]
              tunnel: [w1879] -> w1729
              frame #0 {
                # "④"
                # "setting.iniファイルからの設定項目の読み取り"
                n399 = for {
                  tunnel: "設定12" -> [w1751]
                  tunnel: string[] ["規格", "規格上限", "規格下限", "ポートNo.", "測定モード", "規格単位", "品質チェック項目", "測定周期", "実測MAX", "実測MIN", "実測(MAX)", "実測(MIN)", "測定画面表示ボタン", "ゲージポートNo.", ""] -> [w1746] mode=indexing
                  tunnel: w1738 -> [w1748]
                  tunnel: [w1747] -> w1742
                  tunnel: w1739 -> [w1752]
                  tunnel: [w1750] -> w1743
                  i -> [w1749]
                  n400 = local read "メイン設定_設定 12"() -> (w1744:T1)
                  n401 = case shown="1" w1749 {
                    tunnel: w1752 -> [w1761 w1770 w1779 w1788 w1797 w1806 w1815 w1824 w1833 w1842 w1851 w1860 w1869 w1878]
                    tunnel: [w1760 w1769 w1778 w1787 w1796 w1805 w1814 w1823 w1832 w1841 w1850 w1859 w1868 w1877] -> w1750
                    tunnel: w1751 -> [w1759 w1768 w1777 w1786 w1795 w1804 w1813 w1822 w1831 w1840 w1849 w1858 w1867 w1876]
                    tunnel: w1748 -> [w1758 w1767 w1776 w1785 w1794 w1803 w1812 w1821 w1830 w1839 w1848 w1857 w1866 w1875]
                    tunnel: [w1757 w1766 w1775 w1784 w1793 w1802 w1811 w1820 w1829 w1838 w1847 w1856 w1865 w1874] -> w1747
                    tunnel: w1746 -> [w1755 w1764 w1773 w1782 w1791 w1800 w1809 w1818 w1827 w1836 w1845 w1854 w1863 w1872]
                    tunnel: [w1754 w1763 w1772 w1781 w1790 w1798 w1807 w1816 w1826 w1835 w1844 w1853 w1862 w1871] -> w1745
                    tunnel: w1744 -> [w1753 w1762 w1771 w1780 w1789 w1799 w1808 w1817 w1825 w1834 w1843 w1852 w1861 w1870]
                    frame 0, Default {
                      n402 = call-poly <vilib>:"Read Key.vi"("section"=w1759, "error in (no error)"=w1758, "key"=w1755, "refnum"=w1761) -> ("error out"=w1757:errorcluster, "value"=w1756:string, "refnum out"=w1760:T2)  [unwired: 4 in, 1 out]
                      n403 = Bundle By Name(cluster=w1753, "規格"=w1756) -> (w1754:T1)
                    }
                    frame 1 {
                      n404 = call-poly <vilib>:"Read Key.vi"("section"=w1768, "error in (no error)"=w1767, "key"=w1764, "refnum"=w1770) -> ("error out"=w1766:errorcluster, "value"=w1765:string, "refnum out"=w1769:T2)  [unwired: 4 in, 1 out]
                      n405 = Bundle By Name(cluster=w1762, "規格上限"=w1765) -> (w1763:T1)
                    }
                    frame 2 {
                      n406 = call-poly <vilib>:"Read Key.vi"("section"=w1777, "error in (no error)"=w1776, "key"=w1773, "refnum"=w1779) -> ("error out"=w1775:errorcluster, "value"=w1774:string, "refnum out"=w1778:T2)  [unwired: 4 in, 1 out]
                      n407 = Bundle By Name(cluster=w1771, "規格下限"=w1774) -> (w1772:T1)
                    }
                    frame 3 {
                      n408 = call-poly <vilib>:"Read Key.vi"("section"=w1786, "error in (no error)"=w1785, "key"=w1782, "refnum"=w1788) -> ("error out"=w1784:errorcluster, "value"=w1783:i32, "refnum out"=w1787:T2)  [unwired: 4 in, 1 out]
                      n409 = Bundle By Name(cluster=w1780, "ポートNo."=w1783) -> (w1781:T1)
                    }
                    frame 4 {
                      n410 = call-poly <vilib>:"Read Key.vi"("section"=w1795, "error in (no error)"=w1794, "key"=w1791, "refnum"=w1797) -> ("error out"=w1793:errorcluster, "value"=w1792:i32, "refnum out"=w1796:T2)  [unwired: 4 in, 1 out]
                      n411 = Bundle By Name(cluster=w1789, "測定モード"=w1792) -> (w1790:T1)
                    }
                    frame 5 {
                      n412 = call-poly <vilib>:"Read Key.vi"("section"=w1804, "error in (no error)"=w1803, "key"=w1800, "refnum"=w1806) -> ("error out"=w1802:errorcluster, "value"=w1801:string, "refnum out"=w1805:T2)  [unwired: 4 in, 1 out]
                      n413 = Bundle By Name(cluster=w1799, "規格単位"=w1801) -> (w1798:T1)
                    }
                    frame 6 {
                      n414 = call-poly <vilib>:"Read Key.vi"("section"=w1813, "error in (no error)"=w1812, "key"=w1809, "refnum"=w1815) -> ("error out"=w1811:errorcluster, "value"=w1810:string, "refnum out"=w1814:T2)  [unwired: 4 in, 1 out]
                      n415 = Bundle By Name(cluster=w1808, "品質チェック項目"=w1810) -> (w1807:T1)
                    }
                    frame 7 {
                      n416 = call-poly <vilib>:"Read Key.vi"("section"=w1822, "error in (no error)"=w1821, "key"=w1818, "refnum"=w1824) -> ("error out"=w1820:errorcluster, "value"=w1819:i32, "refnum out"=w1823:T2)  [unwired: 4 in, 1 out]
                      n417 = Bundle By Name(cluster=w1817, "測定周期"=w1819) -> (w1816:T1)
                    }
                    frame 8 {
                      n418 = call-poly <vilib>:"Read Key.vi"("section"=w1831, "error in (no error)"=w1830, "key"=w1827, "refnum"=w1833) -> ("error out"=w1829:errorcluster, "value"=w1828:string, "refnum out"=w1832:T2)  [unwired: 4 in, 1 out]
                      n419 = Bundle By Name(cluster=w1825, "実測値MAX"=w1828) -> (w1826:T1)
                    }
                    frame 9 {
                      n420 = call-poly <vilib>:"Read Key.vi"("section"=w1840, "error in (no error)"=w1839, "key"=w1836, "refnum"=w1842) -> ("error out"=w1838:errorcluster, "value"=w1837:string, "refnum out"=w1841:T2)  [unwired: 4 in, 1 out]
                      n421 = Bundle By Name(cluster=w1834, "実測値MIN"=w1837) -> (w1835:T1)
                    }
                    frame 10 {
                      n422 = call-poly <vilib>:"Read Key.vi"("section"=w1849, "error in (no error)"=w1848, "key"=w1845, "refnum"=w1851) -> ("error out"=w1847:errorcluster, "value"=w1846:string, "refnum out"=w1850:T2)  [unwired: 4 in, 1 out]
                      n423 = Bundle By Name(cluster=w1843, "実測値(MAX)"=w1846) -> (w1844:T1)
                    }
                    frame 11 {
                      n424 = call-poly <vilib>:"Read Key.vi"("section"=w1858, "error in (no error)"=w1857, "key"=w1854, "refnum"=w1860) -> ("error out"=w1856:errorcluster, "value"=w1855:string, "refnum out"=w1859:T2)  [unwired: 4 in, 1 out]
                      n425 = Bundle By Name(cluster=w1852, "実測値(MIN)"=w1855) -> (w1853:T1)
                    }
                    frame 12 {
                      n426 = call-poly <vilib>:"Read Key.vi"("section"=w1867, "error in (no error)"=w1866, "key"=w1863, "refnum"=w1869) -> ("error out"=w1865:errorcluster, "value"=w1864:bool, "refnum out"=w1868:T2)  [unwired: 4 in, 1 out]
                      n427 = Bundle By Name(cluster=w1861, "測定画面表示ボタン"=w1864) -> (w1862:T1)
                    }
                    frame 13 {
                      n428 = call-poly <vilib>:"Read Key.vi"("section"=w1876, "error in (no error)"=w1875, "key"=w1872, "refnum"=w1878) -> ("error out"=w1874:errorcluster, "value"=w1873:string, "refnum out"=w1877:T2)  [unwired: 4 in, 1 out]
                      n429 = Bundle By Name(cluster=w1870, "ゲージポートNo"=w1873) -> (w1871:T1)
                    }
                  }
                  n430 = local write "メイン設定_設定 12"(w1745) -> ()
                }
              }
              frame #1 {
                n431 = local read "メイン設定_設定 12"() -> (w1879:T1)
              }
            }
            n432 = Replace Array Subset(array=w1731, new element=w1729, index=11) -> (w1730:T1[])
          }
          frame 12 {
          }
        }
        n433 = call <vilib>:"Close Config Data.vi"("error in (no error)"=w15, "refnum"=w16) -> ("error out"=→"setup.iniエラーout":errorcluster)  [unwired: 1 in, 8 out]
      }
      n434 = local read "ゲージ確認ボタンBOOL"() -> (w10:bool)
      n435 = Select(t="値転記用配列_\n設定項目画面からの転記", s=w10, f=w9) -> (s? t:f=→"実測設定項目配列_\nメインからの転記":T1[])
    }
    frame #2 {
      # "メインviから設定項目を転記"
      n436 = for {
        N: 32 -> [_]
        i -> [w1889]
        n437 = global read "測定データ転記.vi" "測定転記一時データ"() -> (w1891:string[])
        n438 = Insert Into Array(array=w1891, index=w1889, new element=string[] [""] ("測定転記一時データ")) -> (w1892:string[])
        n439 = global write "測定データ転記.vi" "測定転記一時データ"(w1892) -> ()
      }
      n440 = Wait (ms)(milliseconds to wait=1) -> ()  [unwired: 1 out]
    }
    frame #3 {
      w1893 = 11
      w1910 = 10
      w1911 = 9
      w1928 = 8
      w1929 = 7
      w1946 = 6
      w1947 = 5
      w1964 = 4
      w1965 = 3
      w1974 = 2
      w1982 = 1
      w1990 = 0
      # "メインviから転記された配列のゲージポートNoが空だったらTrue、選択をされていたらFalseを返し処理"
      # "トンネルモード\n最後の値"
      n441 = property on="実測設定項目配列_\nメインからの転記" class="Arr (指定)"() -> ("Value"=w1943:T1[])  [unwired: 2 in, 2 out]
      n442 = property on="実測設定項目配列_\nメインからの転記" class="Arr (指定)"() -> ("Value"=w1932:T1[])  [unwired: 2 in, 2 out]
      n443 = property on="実測設定項目配列_\nメインからの転記" class="Arr (指定)"() -> ("Value"=w1925:T1[])  [unwired: 2 in, 2 out]
      n444 = property on="実測設定項目配列_\nメインからの転記" class="Arr (指定)"() -> ("Value"=w1896:T1[])  [unwired: 2 in, 2 out]
      n445 = property on="実測設定項目配列_\nメインからの転記" class="Arr (指定)"() -> ("Value"=w1968:T1[])  [unwired: 2 in, 2 out]
      n446 = property on="実測設定項目配列_\nメインからの転記" class="Arr (指定)"() -> ("Value"=w1961:T1[])  [unwired: 2 in, 2 out]
      n447 = property on="実測設定項目配列_\nメインからの転記" class="Arr (指定)"() -> ("Value"=w1950:T1[])  [unwired: 2 in, 2 out]
      n448 = property on="実測設定項目配列_\nメインからの転記" class="Arr (指定)"() -> ("Value"=w1907:T1[])  [unwired: 2 in, 2 out]
      n449 = property on="実測設定項目配列_\nメインからの転記" class="Arr (指定)"() -> ("Value"=w1981:T1[])  [unwired: 2 in, 2 out]
      n450 = property on="実測設定項目配列_\nメインからの転記" class="Arr (指定)"() -> ("Value"=w1914:T1[])  [unwired: 2 in, 2 out]
      n451 = property on="実測設定項目配列_\nメインからの転記" class="Arr (指定)"() -> ("Value"=w2001:T1[])  [unwired: 2 in, 2 out]
      n452 = property on="実測設定項目配列_\nメインからの転記" class="Arr (指定)"() -> ("Value"=w1984:T1[])  [unwired: 2 in, 2 out]
      n453 = Index Array(array=w1943, index=w1946) -> (element=w1942:T1)
      n454 = Index Array(array=w1932, index=w1929) -> (element=w1933:T1)
      n455 = Index Array(array=w1925, index=w1928) -> (element=w1924:T1)
      n456 = Index Array(array=w1896, index=w1893) -> (element=w1897:T1)
      n457 = Index Array(array=w1968, index=w1965) -> (element=w1969:T1)
      n458 = Index Array(array=w1961, index=w1964) -> (element=w1960:T1)
      n459 = Index Array(array=w1950, index=w1947) -> (element=w1951:T1)
      n460 = Index Array(array=w1907, index=w1910) -> (element=w1906:T1)
      n461 = Index Array(array=w1981, index=w1974) -> (element=w1980:T1)
      n462 = Index Array(array=w1914, index=w1911) -> (element=w1915:T1)
      n463 = Index Array(array=w2001, index=w1990) -> (element=w2000:T1)
      n464 = Index Array(array=w1984, index=w1982) -> (element=w1985:T1)
      n465 = Unbundle By Name(w1942) -> ("ゲージポートNo"=w1939:refnum<visa-resource-name>)
      n466 = Unbundle By Name(w1933) -> ("ゲージポートNo"=w1936:refnum<visa-resource-name>)
      n467 = Unbundle By Name(w1924) -> ("ゲージポートNo"=w1921:refnum<visa-resource-name>)
      n468 = Unbundle By Name(w1897) -> ("ゲージポートNo"=w1900:refnum<visa-resource-name>)
      n469 = Unbundle By Name(w1969) -> ("ゲージポートNo"=w1972:refnum<visa-resource-name>)
      n470 = Unbundle By Name(w1960) -> ("ゲージポートNo"=w1957:refnum<visa-resource-name>)
      n471 = Unbundle By Name(w1951) -> ("ゲージポートNo"=w1954:refnum<visa-resource-name>)
      n472 = Unbundle By Name(w1906) -> ("ゲージポートNo"=w1903:refnum<visa-resource-name>)
      n473 = Unbundle By Name(w1980) -> ("ゲージポートNo"=w1977:refnum<visa-resource-name>)
      n474 = Unbundle By Name(w1915) -> ("ゲージポートNo"=w1918:refnum<visa-resource-name>)
      n475 = Unbundle By Name(w2000) -> ("ゲージポートNo"=w1993:refnum<visa-resource-name>)
      n476 = Unbundle By Name(w1985) -> ("ゲージポートNo"=w1988:refnum<visa-resource-name>)
      n477 = Empty String/Path?(string/path=w1939) -> (empty?=w1938:bool)
      n478 = Empty String/Path?(string/path=w1936) -> (empty?=w1937:bool)
      n479 = Empty String/Path?(string/path=w1921) -> (empty?=w1920:bool)
      n480 = Empty String/Path?(string/path=w1900) -> (empty?=w1901:bool)
      n481 = Empty String/Path?(string/path=w1972) -> (empty?=w1973:bool)
      n482 = Empty String/Path?(string/path=w1957) -> (empty?=w1956:bool)
      n483 = Empty String/Path?(string/path=w1954) -> (empty?=w1955:bool)
      n484 = Empty String/Path?(string/path=w1903) -> (empty?=w1902:bool)
      n485 = Empty String/Path?(string/path=w1977) -> (empty?=w1976:bool)
      n486 = Empty String/Path?(string/path=w1918) -> (empty?=w1919:bool)
      n487 = Empty String/Path?(string/path=w1993) -> (empty?=w1992:bool)
      n488 = Empty String/Path?(string/path=w1988) -> (empty?=w1989:bool)
      n489 = case shown="TRUE" w1938 {
        tunnel: [w2137 _] -> w1940
        tunnel: w1939 -> [w2140 _]
        tunnel: w1946 -> [_ w2145]
        tunnel: w1946 -> [_ w2144]
        tunnel: w1946 -> [_ w2143]
        frame False {
          n490 = VISA Open(VISA resource name=w2140) -> (VISA resource name=w2138:refnum<visa-resource-name>, error out=w2139:errorcluster)  [unwired: 4 in]
          n491 = case shown="エラーなし" w2139 {
            tunnel: w2138 -> [w2141 w2142]
            tunnel: [w2141 _] -> w2137
            frame No Error {
            }
            frame Error {
              n492 = VISA Close(VISA resource name=w2142) -> ()  [unwired: 1 in, 1 out]
            }
          }
        }
        frame True {
          n493 = for {
            N: 1 -> [_]
            tunnel: w2145 -> [w2149]
            tunnel: w2144 -> [w2148]
            tunnel: w2143 -> [w2147]
            i -> [w2150]
            n494 = case shown="0, デフォルト" w2150 {
              tunnel: w2149 -> [w2152 _]
              tunnel: w2148 -> [w2151 _]
              tunnel: w2147 -> [_ w2160]
              frame 0, Default {
                n495 = flat-sequence {
                  tunnel: w2152 -> [w2153]
                  tunnel: w2151 -> [w2156]
                  frame #0 {
                    n496 = global read "測定データ転記.vi" "測定転記一時データ"() -> (w2154:string[])
                    n497 = Delete From Array(array=w2154, index=w2153) -> (array with subset deleted=w2155:string[])  [unwired: 1 in, 1 out]
                    n498 = global write "測定データ転記.vi" "測定転記一時データ"(w2155) -> ()
                  }
                  frame #1 {
                    n499 = global read "測定データ転記.vi" "測定転記一時データ"() -> (w2159:string[])
                    n500 = Insert Into Array(array=w2159, index=w2156, new element="") -> (w2158:string[])
                    n501 = global write "測定データ転記.vi" "測定転記一時データ"(w2158) -> ()
                  }
                }
              }
              frame 1.. {
                n502 = global read "測定データ転記.vi" "測定転記一時データ"() -> (w2163:string[])
                n503 = Replace Array Subset(array=w2163, new element="", index=w2160) -> (w2162:string[])
                n504 = global write "測定データ転記.vi" "測定転記一時データ"(w2162) -> ()
              }
            }
          }
        }
      }
      n505 = case shown="TRUE" w1937 {
        tunnel: [w2110 _] -> w1935
        tunnel: w1936 -> [w2113 _]
        tunnel: w1929 -> [_ w2118]
        tunnel: w1929 -> [_ w2117]
        tunnel: w1929 -> [_ w2116]
        frame False {
          n506 = VISA Open(VISA resource name=w2113) -> (VISA resource name=w2111:refnum<visa-resource-name>, error out=w2112:errorcluster)  [unwired: 4 in]
          n507 = case shown="エラーなし" w2112 {
            tunnel: w2111 -> [w2114 w2115]
            tunnel: [w2114 _] -> w2110
            frame No Error {
            }
            frame Error {
              n508 = VISA Close(VISA resource name=w2115) -> ()  [unwired: 1 in, 1 out]
            }
          }
        }
        frame True {
          n509 = for {
            N: 1 -> [_]
            tunnel: w2118 -> [w2122]
            tunnel: w2117 -> [w2121]
            tunnel: w2116 -> [w2120]
            i -> [w2123]
            n510 = case shown="0, デフォルト" w2123 {
              tunnel: w2122 -> [w2125 _]
              tunnel: w2121 -> [w2124 _]
              tunnel: w2120 -> [_ w2133]
              frame 0, Default {
                n511 = flat-sequence {
                  tunnel: w2125 -> [w2126]
                  tunnel: w2124 -> [w2129]
                  frame #0 {
                    n512 = global read "測定データ転記.vi" "測定転記一時データ"() -> (w2127:string[])
                    n513 = Delete From Array(array=w2127, index=w2126) -> (array with subset deleted=w2128:string[])  [unwired: 1 in, 1 out]
                    n514 = global write "測定データ転記.vi" "測定転記一時データ"(w2128) -> ()
                  }
                  frame #1 {
                    n515 = global read "測定データ転記.vi" "測定転記一時データ"() -> (w2132:string[])
                    n516 = Insert Into Array(array=w2132, index=w2129, new element="") -> (w2131:string[])
                    n517 = global write "測定データ転記.vi" "測定転記一時データ"(w2131) -> ()
                  }
                }
              }
              frame 1.. {
                n518 = global read "測定データ転記.vi" "測定転記一時データ"() -> (w2136:string[])
                n519 = Replace Array Subset(array=w2136, new element="", index=w2133) -> (w2135:string[])
                n520 = global write "測定データ転記.vi" "測定転記一時データ"(w2135) -> ()
              }
            }
          }
        }
      }
      n521 = case shown="TRUE" w1920 {
        tunnel: [w2083 _] -> w1922
        tunnel: w1921 -> [w2086 _]
        tunnel: w1928 -> [_ w2091]
        tunnel: w1928 -> [_ w2090]
        tunnel: w1928 -> [_ w2089]
        frame False {
          n522 = VISA Open(VISA resource name=w2086) -> (VISA resource name=w2084:refnum<visa-resource-name>, error out=w2085:errorcluster)  [unwired: 4 in]
          n523 = case shown="エラーなし" w2085 {
            tunnel: w2084 -> [w2087 w2088]
            tunnel: [w2087 _] -> w2083
            frame No Error {
            }
            frame Error {
              n524 = VISA Close(VISA resource name=w2088) -> ()  [unwired: 1 in, 1 out]
            }
          }
        }
        frame True {
          n525 = for {
            N: 1 -> [_]
            tunnel: w2091 -> [w2095]
            tunnel: w2090 -> [w2094]
            tunnel: w2089 -> [w2093]
            i -> [w2096]
            n526 = case shown="0, デフォルト" w2096 {
              tunnel: w2095 -> [w2098 _]
              tunnel: w2094 -> [w2097 _]
              tunnel: w2093 -> [_ w2106]
              frame 0, Default {
                n527 = flat-sequence {
                  tunnel: w2098 -> [w2099]
                  tunnel: w2097 -> [w2102]
                  frame #0 {
                    n528 = global read "測定データ転記.vi" "測定転記一時データ"() -> (w2100:string[])
                    n529 = Delete From Array(array=w2100, index=w2099) -> (array with subset deleted=w2101:string[])  [unwired: 1 in, 1 out]
                    n530 = global write "測定データ転記.vi" "測定転記一時データ"(w2101) -> ()
                  }
                  frame #1 {
                    n531 = global read "測定データ転記.vi" "測定転記一時データ"() -> (w2105:string[])
                    n532 = Insert Into Array(array=w2105, index=w2102, new element="") -> (w2104:string[])
                    n533 = global write "測定データ転記.vi" "測定転記一時データ"(w2104) -> ()
                  }
                }
              }
              frame 1.. {
                n534 = global read "測定データ転記.vi" "測定転記一時データ"() -> (w2109:string[])
                n535 = Replace Array Subset(array=w2109, new element="", index=w2106) -> (w2108:string[])
                n536 = global write "測定データ転記.vi" "測定転記一時データ"(w2108) -> ()
              }
            }
          }
        }
      }
      n537 = case shown="TRUE" w1901 {
        tunnel: [w2002 _] -> w1899
        tunnel: w1900 -> [w2005 _]
        tunnel: w1893 -> [_ w2010]
        tunnel: w1893 -> [_ w2009]
        tunnel: w1893 -> [_ w2008]
        frame False {
          n538 = VISA Open(VISA resource name=w2005) -> (VISA resource name=w2003:refnum<visa-resource-name>, error out=w2004:errorcluster)  [unwired: 4 in]
          n539 = case shown="エラーなし" w2004 {
            tunnel: w2003 -> [w2006 w2007]
            tunnel: [w2006 _] -> w2002
            frame No Error {
            }
            frame Error {
              n540 = VISA Close(VISA resource name=w2007) -> ()  [unwired: 1 in, 1 out]
            }
          }
        }
        frame True {
          n541 = for {
            N: 1 -> [_]
            tunnel: w2010 -> [w2014]
            tunnel: w2009 -> [w2013]
            tunnel: w2008 -> [w2012]
            i -> [w2015]
            n542 = case shown="0, デフォルト" w2015 {
              tunnel: w2014 -> [w2017 _]
              tunnel: w2013 -> [w2016 _]
              tunnel: w2012 -> [_ w2025]
              frame 0, Default {
                n543 = flat-sequence {
                  tunnel: w2017 -> [w2018]
                  tunnel: w2016 -> [w2021]
                  frame #0 {
                    n544 = global read "測定データ転記.vi" "測定転記一時データ"() -> (w2019:string[])
                    n545 = Delete From Array(array=w2019, index=w2018) -> (array with subset deleted=w2020:string[])  [unwired: 1 in, 1 out]
                    n546 = global write "測定データ転記.vi" "測定転記一時データ"(w2020) -> ()
                  }
                  frame #1 {
                    n547 = global read "測定データ転記.vi" "測定転記一時データ"() -> (w2024:string[])
                    n548 = Insert Into Array(array=w2024, index=w2021, new element="") -> (w2023:string[])
                    n549 = global write "測定データ転記.vi" "測定転記一時データ"(w2023) -> ()
                  }
                }
              }
              frame 1.. {
                n550 = global read "測定データ転記.vi" "測定転記一時データ"() -> (w2028:string[])
                n551 = Replace Array Subset(array=w2028, new element="", index=w2025) -> (w2027:string[])
                n552 = global write "測定データ転記.vi" "測定転記一時データ"(w2027) -> ()
              }
            }
          }
        }
      }
      n553 = case shown="TRUE" w1973 {
        tunnel: [w2218 _] -> w1971
        tunnel: w1972 -> [w2221 _]
        tunnel: w1965 -> [_ w2226]
        tunnel: w1965 -> [_ w2225]
        tunnel: w1965 -> [_ w2224]
        frame False {
          n554 = VISA Open(VISA resource name=w2221) -> (VISA resource name=w2219:refnum<visa-resource-name>, error out=w2220:errorcluster)  [unwired: 4 in]
          n555 = case shown="エラーなし" w2220 {
            tunnel: w2219 -> [w2222 w2223]
            tunnel: [w2222 _] -> w2218
            frame No Error {
            }
            frame Error {
              n556 = VISA Close(VISA resource name=w2223) -> ()  [unwired: 1 in, 1 out]
            }
          }
        }
        frame True {
          n557 = for {
            N: 1 -> [_]
            tunnel: w2226 -> [w2230]
            tunnel: w2225 -> [w2229]
            tunnel: w2224 -> [w2228]
            i -> [w2231]
            n558 = case shown="0, デフォルト" w2231 {
              tunnel: w2230 -> [w2233 _]
              tunnel: w2229 -> [w2232 _]
              tunnel: w2228 -> [_ w2241]
              frame 0, Default {
                n559 = flat-sequence {
                  tunnel: w2233 -> [w2234]
                  tunnel: w2232 -> [w2237]
                  frame #0 {
                    n560 = global read "測定データ転記.vi" "測定転記一時データ"() -> (w2235:string[])
                    n561 = Delete From Array(array=w2235, index=w2234) -> (array with subset deleted=w2236:string[])  [unwired: 1 in, 1 out]
                    n562 = global write "測定データ転記.vi" "測定転記一時データ"(w2236) -> ()
                  }
                  frame #1 {
                    n563 = global read "測定データ転記.vi" "測定転記一時データ"() -> (w2240:string[])
                    n564 = Insert Into Array(array=w2240, index=w2237, new element="") -> (w2239:string[])
                    n565 = global write "測定データ転記.vi" "測定転記一時データ"(w2239) -> ()
                  }
                }
              }
              frame 1.. {
                n566 = global read "測定データ転記.vi" "測定転記一時データ"() -> (w2244:string[])
                n567 = Replace Array Subset(array=w2244, new element="", index=w2241) -> (w2243:string[])
                n568 = global write "測定データ転記.vi" "測定転記一時データ"(w2243) -> ()
              }
            }
          }
        }
      }
      n569 = case shown="TRUE" w1956 {
        tunnel: [w2191 _] -> w1958
        tunnel: w1957 -> [w2194 _]
        tunnel: w1964 -> [_ w2199]
        tunnel: w1964 -> [_ w2198]
        tunnel: w1964 -> [_ w2197]
        frame False {
          n570 = VISA Open(VISA resource name=w2194) -> (VISA resource name=w2192:refnum<visa-resource-name>, error out=w2193:errorcluster)  [unwired: 4 in]
          n571 = case shown="エラーなし" w2193 {
            tunnel: w2192 -> [w2195 w2196]
            tunnel: [w2195 _] -> w2191
            frame No Error {
            }
            frame Error {
              n572 = VISA Close(VISA resource name=w2196) -> ()  [unwired: 1 in, 1 out]
            }
          }
        }
        frame True {
          n573 = for {
            N: 1 -> [_]
            tunnel: w2199 -> [w2203]
            tunnel: w2198 -> [w2202]
            tunnel: w2197 -> [w2201]
            i -> [w2204]
            n574 = case shown="0, デフォルト" w2204 {
              tunnel: w2203 -> [w2206 _]
              tunnel: w2202 -> [w2205 _]
              tunnel: w2201 -> [_ w2214]
              frame 0, Default {
                n575 = flat-sequence {
                  tunnel: w2206 -> [w2207]
                  tunnel: w2205 -> [w2210]
                  frame #0 {
                    n576 = global read "測定データ転記.vi" "測定転記一時データ"() -> (w2208:string[])
                    n577 = Delete From Array(array=w2208, index=w2207) -> (array with subset deleted=w2209:string[])  [unwired: 1 in, 1 out]
                    n578 = global write "測定データ転記.vi" "測定転記一時データ"(w2209) -> ()
                  }
                  frame #1 {
                    n579 = global read "測定データ転記.vi" "測定転記一時データ"() -> (w2213:string[])
                    n580 = Insert Into Array(array=w2213, index=w2210, new element="") -> (w2212:string[])
                    n581 = global write "測定データ転記.vi" "測定転記一時データ"(w2212) -> ()
                  }
                }
              }
              frame 1.. {
                n582 = global read "測定データ転記.vi" "測定転記一時データ"() -> (w2217:string[])
                n583 = Replace Array Subset(array=w2217, new element="", index=w2214) -> (w2216:string[])
                n584 = global write "測定データ転記.vi" "測定転記一時データ"(w2216) -> ()
              }
            }
          }
        }
      }
      n585 = case shown="TRUE" w1955 {
        tunnel: [w2164 _] -> w1953
        tunnel: w1954 -> [w2167 _]
        tunnel: w1947 -> [_ w2172]
        tunnel: w1947 -> [_ w2171]
        tunnel: w1947 -> [_ w2170]
        frame False {
          n586 = VISA Open(VISA resource name=w2167) -> (VISA resource name=w2165:refnum<visa-resource-name>, error out=w2166:errorcluster)  [unwired: 4 in]
          n587 = case shown="エラーなし" w2166 {
            tunnel: w2165 -> [w2168 w2169]
            tunnel: [w2168 _] -> w2164
            frame No Error {
            }
            frame Error {
              n588 = VISA Close(VISA resource name=w2169) -> ()  [unwired: 1 in, 1 out]
            }
          }
        }
        frame True {
          n589 = for {
            N: 1 -> [_]
            tunnel: w2172 -> [w2176]
            tunnel: w2171 -> [w2175]
            tunnel: w2170 -> [w2174]
            i -> [w2177]
            n590 = case shown="0, デフォルト" w2177 {
              tunnel: w2176 -> [w2179 _]
              tunnel: w2175 -> [w2178 _]
              tunnel: w2174 -> [_ w2187]
              frame 0, Default {
                n591 = flat-sequence {
                  tunnel: w2179 -> [w2180]
                  tunnel: w2178 -> [w2183]
                  frame #0 {
                    n592 = global read "測定データ転記.vi" "測定転記一時データ"() -> (w2181:string[])
                    n593 = Delete From Array(array=w2181, index=w2180) -> (array with subset deleted=w2182:string[])  [unwired: 1 in, 1 out]
                    n594 = global write "測定データ転記.vi" "測定転記一時データ"(w2182) -> ()
                  }
                  frame #1 {
                    n595 = global read "測定データ転記.vi" "測定転記一時データ"() -> (w2186:string[])
                    n596 = Insert Into Array(array=w2186, index=w2183, new element="") -> (w2185:string[])
                    n597 = global write "測定データ転記.vi" "測定転記一時データ"(w2185) -> ()
                  }
                }
              }
              frame 1.. {
                n598 = global read "測定データ転記.vi" "測定転記一時データ"() -> (w2190:string[])
                n599 = Replace Array Subset(array=w2190, new element="", index=w2187) -> (w2189:string[])
                n600 = global write "測定データ転記.vi" "測定転記一時データ"(w2189) -> ()
              }
            }
          }
        }
      }
      n601 = case shown="TRUE" w1902 {
        tunnel: [w2029 _] -> w1904
        tunnel: w1903 -> [w2032 _]
        tunnel: w1910 -> [_ w2037]
        tunnel: w1910 -> [_ w2036]
        tunnel: w1910 -> [_ w2035]
        frame False {
          n602 = VISA Open(VISA resource name=w2032) -> (VISA resource name=w2030:refnum<visa-resource-name>, error out=w2031:errorcluster)  [unwired: 4 in]
          n603 = case shown="エラーなし" w2031 {
            tunnel: w2030 -> [w2033 w2034]
            tunnel: [w2033 _] -> w2029
            frame No Error {
            }
            frame Error {
              n604 = VISA Close(VISA resource name=w2034) -> ()  [unwired: 1 in, 1 out]
            }
          }
        }
        frame True {
          n605 = for {
            N: 1 -> [_]
            tunnel: w2037 -> [w2041]
            tunnel: w2036 -> [w2040]
            tunnel: w2035 -> [w2039]
            i -> [w2042]
            n606 = case shown="0, デフォルト" w2042 {
              tunnel: w2041 -> [w2044 _]
              tunnel: w2040 -> [w2043 _]
              tunnel: w2039 -> [_ w2052]
              frame 0, Default {
                n607 = flat-sequence {
                  tunnel: w2044 -> [w2045]
                  tunnel: w2043 -> [w2048]
                  frame #0 {
                    n608 = global read "測定データ転記.vi" "測定転記一時データ"() -> (w2046:string[])
                    n609 = Delete From Array(array=w2046, index=w2045) -> (array with subset deleted=w2047:string[])  [unwired: 1 in, 1 out]
                    n610 = global write "測定データ転記.vi" "測定転記一時データ"(w2047) -> ()
                  }
                  frame #1 {
                    n611 = global read "測定データ転記.vi" "測定転記一時データ"() -> (w2051:string[])
                    n612 = Insert Into Array(array=w2051, index=w2048, new element="") -> (w2050:string[])
                    n613 = global write "測定データ転記.vi" "測定転記一時データ"(w2050) -> ()
                  }
                }
              }
              frame 1.. {
                n614 = global read "測定データ転記.vi" "測定転記一時データ"() -> (w2055:string[])
                n615 = Replace Array Subset(array=w2055, new element="", index=w2052) -> (w2054:string[])
                n616 = global write "測定データ転記.vi" "測定転記一時データ"(w2054) -> ()
              }
            }
          }
        }
      }
      n617 = case shown="TRUE" w1976 {
        tunnel: [w2245 _] -> w1978
        tunnel: w1977 -> [w2248 _]
        tunnel: w1974 -> [_ w2253]
        tunnel: w1974 -> [_ w2252]
        tunnel: w1974 -> [_ w2251]
        frame False {
          n618 = VISA Open(VISA resource name=w2248) -> (VISA resource name=w2246:refnum<visa-resource-name>, error out=w2247:errorcluster)  [unwired: 4 in]
          n619 = case shown="エラーなし" w2247 {
            tunnel: w2246 -> [w2249 w2250]
            tunnel: [w2249 _] -> w2245
            frame No Error {
            }
            frame Error {
              n620 = VISA Close(VISA resource name=w2250) -> ()  [unwired: 1 in, 1 out]
            }
          }
        }
        frame True {
          n621 = for {
            N: 1 -> [_]
            tunnel: w2253 -> [w2257]
            tunnel: w2252 -> [w2256]
            tunnel: w2251 -> [w2255]
            i -> [w2258]
            n622 = case shown="0, デフォルト" w2258 {
              tunnel: w2257 -> [w2260 _]
              tunnel: w2256 -> [w2259 _]
              tunnel: w2255 -> [_ w2268]
              frame 0, Default {
                n623 = flat-sequence {
                  tunnel: w2260 -> [w2261]
                  tunnel: w2259 -> [w2264]
                  frame #0 {
                    n624 = global read "測定データ転記.vi" "測定転記一時データ"() -> (w2262:string[])
                    n625 = Delete From Array(array=w2262, index=w2261) -> (array with subset deleted=w2263:string[])  [unwired: 1 in, 1 out]
                    n626 = global write "測定データ転記.vi" "測定転記一時データ"(w2263) -> ()
                  }
                  frame #1 {
                    n627 = global read "測定データ転記.vi" "測定転記一時データ"() -> (w2267:string[])
                    n628 = Insert Into Array(array=w2267, index=w2264, new element="") -> (w2266:string[])
                    n629 = global write "測定データ転記.vi" "測定転記一時データ"(w2266) -> ()
                  }
                }
              }
              frame 1.. {
                n630 = global read "測定データ転記.vi" "測定転記一時データ"() -> (w2271:string[])
                n631 = Replace Array Subset(array=w2271, new element="", index=w2268) -> (w2270:string[])
                n632 = global write "測定データ転記.vi" "測定転記一時データ"(w2270) -> ()
              }
            }
          }
        }
      }
      n633 = case shown="TRUE" w1919 {
        tunnel: [w2056 _] -> w1917
        tunnel: w1918 -> [w2059 _]
        tunnel: w1911 -> [_ w2064]
        tunnel: w1911 -> [_ w2063]
        tunnel: w1911 -> [_ w2062]
        frame False {
          n634 = VISA Open(VISA resource name=w2059) -> (VISA resource name=w2057:refnum<visa-resource-name>, error out=w2058:errorcluster)  [unwired: 4 in]
          n635 = case shown="エラーなし" w2058 {
            tunnel: w2057 -> [w2060 w2061]
            tunnel: [w2060 _] -> w2056
            frame No Error {
            }
            frame Error {
              n636 = VISA Close(VISA resource name=w2061) -> ()  [unwired: 1 in, 1 out]
            }
          }
        }
        frame True {
          n637 = for {
            N: 1 -> [_]
            tunnel: w2064 -> [w2068]
            tunnel: w2063 -> [w2067]
            tunnel: w2062 -> [w2066]
            i -> [w2069]
            n638 = case shown="0, デフォルト" w2069 {
              tunnel: w2068 -> [w2071 _]
              tunnel: w2067 -> [w2070 _]
              tunnel: w2066 -> [_ w2079]
              frame 0, Default {
                n639 = flat-sequence {
                  tunnel: w2071 -> [w2072]
                  tunnel: w2070 -> [w2075]
                  frame #0 {
                    n640 = global read "測定データ転記.vi" "測定転記一時データ"() -> (w2073:string[])
                    n641 = Delete From Array(array=w2073, index=w2072) -> (array with subset deleted=w2074:string[])  [unwired: 1 in, 1 out]
                    n642 = global write "測定データ転記.vi" "測定転記一時データ"(w2074) -> ()
                  }
                  frame #1 {
                    n643 = global read "測定データ転記.vi" "測定転記一時データ"() -> (w2078:string[])
                    n644 = Insert Into Array(array=w2078, index=w2075, new element="") -> (w2077:string[])
                    n645 = global write "測定データ転記.vi" "測定転記一時データ"(w2077) -> ()
                  }
                }
              }
              frame 1.. {
                n646 = global read "測定データ転記.vi" "測定転記一時データ"() -> (w2082:string[])
                n647 = Replace Array Subset(array=w2082, new element="", index=w2079) -> (w2081:string[])
                n648 = global write "測定データ転記.vi" "測定転記一時データ"(w2081) -> ()
              }
            }
          }
        }
      }
      n649 = case shown="TRUE" w1992 {
        tunnel: [w2350 _] -> w1997
        tunnel: w1993 -> [w2353 _]
        tunnel: w1990 -> [_ w2358]
        tunnel: w1990 -> [_ w2357]
        tunnel: w1990 -> [_ w2356]
        frame False {
          n650 = VISA Open(VISA resource name=w2353) -> (VISA resource name=w2351:refnum<visa-resource-name>, error out=w2352:errorcluster)  [unwired: 4 in]
          n651 = case shown="エラーなし" w2352 {
            tunnel: w2351 -> [w2354 w2355]
            tunnel: [w2354 _] -> w2350
            frame No Error {
            }
            frame Error {
              n652 = VISA Close(VISA resource name=w2355) -> ()  [unwired: 1 in, 1 out]
            }
          }
        }
        frame True {
          n653 = for {
            N: 1 -> [_]
            tunnel: w2358 -> [w2362]
            tunnel: w2357 -> [w2361]
            tunnel: w2356 -> [w2360]
            i -> [w2363]
            n654 = case shown="0, デフォルト" w2363 {
              tunnel: w2362 -> [w2365 _]
              tunnel: w2361 -> [w2364 _]
              tunnel: w2360 -> [_ w2373]
              frame 0, Default {
                n655 = flat-sequence {
                  tunnel: w2365 -> [w2366]
                  tunnel: w2364 -> [w2369]
                  frame #0 {
                    n656 = global read "測定データ転記.vi" "測定転記一時データ"() -> (w2367:string[])
                    n657 = Delete From Array(array=w2367, index=w2366) -> (array with subset deleted=w2368:string[])  [unwired: 1 in, 1 out]
                    n658 = global write "測定データ転記.vi" "測定転記一時データ"(w2368) -> ()
                  }
                  frame #1 {
                    n659 = global read "測定データ転記.vi" "測定転記一時データ"() -> (w2372:string[])
                    n660 = Insert Into Array(array=w2372, index=w2369, new element="") -> (w2371:string[])
                    n661 = global write "測定データ転記.vi" "測定転記一時データ"(w2371) -> ()
                  }
                }
              }
              frame 1.. {
                n662 = global read "測定データ転記.vi" "測定転記一時データ"() -> (w2376:string[])
                n663 = Replace Array Subset(array=w2376, new element="", index=w2373) -> (w2375:string[])
                n664 = global write "測定データ転記.vi" "測定転記一時データ"(w2375) -> ()
              }
            }
          }
        }
      }
      n665 = case shown="TRUE" w1989 {
        tunnel: [w2272 _] -> w1987
        tunnel: w1988 -> [w2275 _]
        tunnel: w1982 -> [_ w2280]
        tunnel: w1982 -> [_ w2279]
        tunnel: w1982 -> [_ w2278]
        frame False {
          n666 = VISA Open(VISA resource name=w2275) -> (VISA resource name=w2273:refnum<visa-resource-name>, error out=w2274:errorcluster)  [unwired: 4 in]
          n667 = case shown="エラーなし" w2274 {
            tunnel: w2273 -> [w2276 w2277]
            tunnel: [w2276 _] -> w2272
            frame No Error {
            }
            frame Error {
              n668 = VISA Close(VISA resource name=w2277) -> ()  [unwired: 1 in, 1 out]
            }
          }
        }
        frame True {
          n669 = for {
            N: 1 -> [_]
            tunnel: w2280 -> [w2284]
            tunnel: w2279 -> [w2283]
            tunnel: w2278 -> [w2282]
            i -> [w2285]
            n670 = case shown="0, デフォルト" w2285 {
              tunnel: w2284 -> [w2287 _]
              tunnel: w2283 -> [w2286 _]
              tunnel: w2282 -> [_ w2295]
              frame 0, Default {
                n671 = flat-sequence {
                  tunnel: w2287 -> [w2288]
                  tunnel: w2286 -> [w2291]
                  frame #0 {
                    n672 = global read "測定データ転記.vi" "測定転記一時データ"() -> (w2289:string[])
                    n673 = Delete From Array(array=w2289, index=w2288) -> (array with subset deleted=w2290:string[])  [unwired: 1 in, 1 out]
                    n674 = global write "測定データ転記.vi" "測定転記一時データ"(w2290) -> ()
                  }
                  frame #1 {
                    n675 = global read "測定データ転記.vi" "測定転記一時データ"() -> (w2294:string[])
                    n676 = Insert Into Array(array=w2294, index=w2291, new element="") -> (w2293:string[])
                    n677 = global write "測定データ転記.vi" "測定転記一時データ"(w2293) -> ()
                  }
                }
              }
              frame 1.. {
                n678 = global read "測定データ転記.vi" "測定転記一時データ"() -> (w2298:string[])
                n679 = Replace Array Subset(array=w2298, new element="", index=w2295) -> (w2297:string[])
                n680 = global write "測定データ転記.vi" "測定転記一時データ"(w2297) -> ()
              }
            }
          }
        }
      }
      n681 = property class="Instr"(reference=w1940, "TermChar"=u8 13 ("Message Based Settings:Termination Character")) -> (reference out=w1945:refnum<visa-resource-name>)  [unwired: 1 in, 1 out]
      n682 = property class="Instr"(reference=w1935, "TermChar"=u8 13 ("Message Based Settings:Termination Character")) -> (reference out=w1930:refnum<visa-resource-name>)  [unwired: 1 in, 1 out]
      n683 = property class="Instr"(reference=w1922, "TermChar"=u8 13 ("Message Based Settings:Termination Character")) -> (reference out=w1927:refnum<visa-resource-name>)  [unwired: 1 in, 1 out]
      n684 = property class="Instr"(reference=w1899, "TermChar"=u8 13 ("Message Based Settings:Termination Character")) -> (reference out=w1894:refnum<visa-resource-name>)  [unwired: 1 in, 1 out]
      n685 = property class="Instr"(reference=w1971, "TermChar"=u8 13 ("Message Based Settings:Termination Character")) -> (reference out=w1966:refnum<visa-resource-name>)  [unwired: 1 in, 1 out]
      n686 = property class="Instr"(reference=w1958, "TermChar"=u8 13 ("Message Based Settings:Termination Character")) -> (reference out=w1963:refnum<visa-resource-name>)  [unwired: 1 in, 1 out]
      n687 = property class="Instr"(reference=w1953, "TermChar"=u8 13 ("Message Based Settings:Termination Character")) -> (reference out=w1948:refnum<visa-resource-name>)  [unwired: 1 in, 1 out]
      n688 = property class="Instr"(reference=w1904, "TermChar"=u8 13 ("Message Based Settings:Termination Character")) -> (reference out=w1909:refnum<visa-resource-name>)  [unwired: 1 in, 1 out]
      n689 = property class="Instr"(reference=w1978, "TermChar"=u8 13 ("Message Based Settings:Termination Character")) -> (reference out=w1975:refnum<visa-resource-name>)  [unwired: 1 in, 1 out]
      n690 = property class="Instr"(reference=w1917, "TermChar"=u8 13 ("Message Based Settings:Termination Character")) -> (reference out=w1912:refnum<visa-resource-name>)  [unwired: 1 in, 1 out]
      n691 = property class="Instr"(reference=w1997, "TermChar"=u8 13 ("Message Based Settings:Termination Character")) -> (reference out=w1999:refnum<visa-resource-name>)  [unwired: 1 in, 1 out]
      n692 = property class="Instr"(reference=w1987, "TermChar"=u8 13 ("Message Based Settings:Termination Character")) -> (reference out=w1983:refnum<visa-resource-name>)  [unwired: 1 in, 1 out]
      n693 = while {
        tunnel: w1999 -> [w2349]
        tunnel: [w2348] -> w1996
        tunnel: w1983 -> [w2345]
        tunnel: [w2346] -> w1995
        tunnel: w1975 -> [w2342]
        tunnel: [w2343] -> w1994
        tunnel: w1991 -> [w2340]
        tunnel: w1990 -> [w2339]
        tunnel: w1982 -> [w2338]
        tunnel: w1974 -> [w2337]
        tunnel: [w2335] -> w1967
        tunnel: w1966 -> [w2334]
        tunnel: w1965 -> [w2333]
        tunnel: [w2330] -> w1962
        tunnel: w1963 -> [w2331]
        tunnel: w1964 -> [w2332]
        tunnel: [w2327] -> w1949
        tunnel: w1948 -> [w2326]
        tunnel: w1947 -> [w2325]
        tunnel: [w2322] -> w1944
        tunnel: w1945 -> [w2323]
        tunnel: w1946 -> [w2324]
        tunnel: [w2319] -> w1931
        tunnel: w1930 -> [w2318]
        tunnel: w1929 -> [w2317]
        tunnel: [w2314] -> w1926
        tunnel: w1927 -> [w2315]
        tunnel: w1928 -> [w2316]
        tunnel: [w2311] -> w1913
        tunnel: w1912 -> [w2310]
        tunnel: w1911 -> [w2309]
        tunnel: [w2306] -> w1908
        tunnel: w1909 -> [w2307]
        tunnel: w1910 -> [w2308]
        tunnel: [w2303] -> w1895
        tunnel: w1894 -> [w2302]
        tunnel: w1893 -> [w2301]
        i -> [w2300]
        stop <- w2299 stop-if-true
        n694 = call "ゲージデータ取り込み_サブ1.vi"("配列指標"=w2339, "ループ回数数値"=w2300, "VISA Refnum入力"=w2349) -> ("エラー出力"=→"ゲージエラー 1":errorcluster, "VISA Refnum出力"=w2348:refnum<visa-resource-name>)  [unwired: 7 in]
        n695 = call "ゲージデータ取り込み_サブ1.vi"("配列指標"=w2338, "ループ回数数値"=w2300, "VISA Refnum入力"=w2345) -> ("エラー出力"=→"ゲージエラー 2":errorcluster, "VISA Refnum出力"=w2346:refnum<visa-resource-name>)  [unwired: 7 in]
        n696 = global read "VISA停止_G.vi" "VISA停止_\nグローバル"() -> (w2299:bool)
        n697 = call "ゲージデータ取り込み_サブ1.vi"("配列指標"=w2324, "ループ回数数値"=w2300, "VISA Refnum入力"=w2323) -> ("エラー出力"=→"ゲージエラー 7":errorcluster, "VISA Refnum出力"=w2322:refnum<visa-resource-name>)  [unwired: 7 in]
        n698 = call "ゲージデータ取り込み_サブ1.vi"("配列指標"=w2317, "ループ回数数値"=w2300, "VISA Refnum入力"=w2318) -> ("エラー出力"=→"ゲージエラー 8":errorcluster, "VISA Refnum出力"=w2319:refnum<visa-resource-name>)  [unwired: 7 in]
        n699 = call "ゲージデータ取り込み_サブ1.vi"("配列指標"=w2316, "ループ回数数値"=w2300, "VISA Refnum入力"=w2315) -> ("エラー出力"=→"ゲージエラー 9":errorcluster, "VISA Refnum出力"=w2314:refnum<visa-resource-name>)  [unwired: 7 in]
        n700 = call "ゲージデータ取り込み_サブ1.vi"("配列指標"=w2301, "ループ回数数値"=w2300, "VISA Refnum入力"=w2302) -> ("エラー出力"=→"ゲージエラー 12":errorcluster, "VISA Refnum出力"=w2303:refnum<visa-resource-name>)  [unwired: 7 in]
        n701 = call "ゲージデータ取り込み_サブ1.vi"("配列指標"=w2337, "ループ回数数値"=w2300, "VISA Refnum入力"=w2342) -> ("エラー出力"=→"ゲージエラー 3":errorcluster, "VISA Refnum出力"=w2343:refnum<visa-resource-name>)  [unwired: 7 in]
        n702 = call "ゲージデータ取り込み_サブ1.vi"("配列指標"=w2333, "ループ回数数値"=w2300, "VISA Refnum入力"=w2334) -> ("エラー出力"=→"ゲージエラー 4":errorcluster, "VISA Refnum出力"=w2335:refnum<visa-resource-name>)  [unwired: 7 in]
        n703 = call "ゲージデータ取り込み_サブ1.vi"("配列指標"=w2332, "ループ回数数値"=w2300, "VISA Refnum入力"=w2331) -> ("エラー出力"=→"ゲージエラー 5":errorcluster, "VISA Refnum出力"=w2330:refnum<visa-resource-name>)  [unwired: 7 in]
        n704 = call "ゲージデータ取り込み_サブ1.vi"("配列指標"=w2325, "ループ回数数値"=w2300, "VISA Refnum入力"=w2326) -> ("エラー出力"=→"ゲージエラー 6":errorcluster, "VISA Refnum出力"=w2327:refnum<visa-resource-name>)  [unwired: 7 in]
        n705 = call "ゲージデータ取り込み_サブ1.vi"("配列指標"=w2308, "ループ回数数値"=w2300, "VISA Refnum入力"=w2307) -> ("エラー出力"=→"ゲージエラー 11":errorcluster, "VISA Refnum出力"=w2306:refnum<visa-resource-name>)  [unwired: 7 in]
        n706 = call "ゲージデータ取り込み_サブ1.vi"("配列指標"=w2309, "ループ回数数値"=w2300, "VISA Refnum入力"=w2310) -> ("エラー出力"=→"ゲージエラー 10":errorcluster, "VISA Refnum出力"=w2311:refnum<visa-resource-name>)  [unwired: 7 in]
        n707 = Wait Until Next ms Multiple(millisecond multiple=w2340) -> ()  [unwired: 1 out]
      }
      n708 = VISA Close(VISA resource name=w1996) -> ()  [unwired: 1 in, 1 out]
      n709 = VISA Close(VISA resource name=w1944) -> ()  [unwired: 1 in, 1 out]
      n710 = VISA Close(VISA resource name=w1931) -> ()  [unwired: 1 in, 1 out]
      n711 = VISA Close(VISA resource name=w1926) -> ()  [unwired: 1 in, 1 out]
      n712 = VISA Close(VISA resource name=w1895) -> ()  [unwired: 1 in, 1 out]
      n713 = VISA Close(VISA resource name=w1995) -> ()  [unwired: 1 in, 1 out]
      n714 = VISA Close(VISA resource name=w1994) -> ()  [unwired: 1 in, 1 out]
      n715 = VISA Close(VISA resource name=w1967) -> ()  [unwired: 1 in, 1 out]
      n716 = VISA Close(VISA resource name=w1962) -> ()  [unwired: 1 in, 1 out]
      n717 = VISA Close(VISA resource name=w1949) -> ()  [unwired: 1 in, 1 out]
      n718 = VISA Close(VISA resource name=w1908) -> ()  [unwired: 1 in, 1 out]
      n719 = VISA Close(VISA resource name=w1913) -> ()  [unwired: 1 in, 1 out]
    }
    frame #4 {
      # "ゲージ確認ボタンBOOLの初期化"
      n720 = local write "ゲージ確認ボタンBOOL"(FALSE) -> ()
    }
  }
